vi "ArmControlManager.vi"(0 "Arm Shoulder Manual Control":dbl, 1 "Arm Extend Manual Control":dbl, 3 "Shoulder Sensor Unit Conversion (ticks/rad)":dbl, 4 "Extend Sensor Unit Coversion (ticks/in)":dbl, 5 "Arm Shoulder Motion Profile":T22[](array[typedef]) {"Time (ms)" items=["TrajectoryDuration_0ms"=0, "TrajectoryDuration_5ms"=5, "TrajectoryDuration_10ms"=10, "TrajectoryDuration_20ms"=20, "TrajectoryDuration_30ms"=30, "TrajectoryDuration_40ms"=40, "TrajectoryDuration_50ms"=50, "TrajectoryDuration_100ms"=100]}, 7 "Arm Extend Motion Profile":T22[](array[typedef]) {"Time (ms)" items=["TrajectoryDuration_0ms"=0, "TrajectoryDuration_5ms"=5, "TrajectoryDuration_10ms"=10, "TrajectoryDuration_20ms"=20, "TrajectoryDuration_30ms"=30, "TrajectoryDuration_40ms"=40, "TrajectoryDuration_50ms"=50, "TrajectoryDuration_100ms"=100]}, 8 "ArmCompleteNotifier":refnum<notifier>, 9 "Arm Wrist Motion Profile":T22[](array[typedef]) {"Time (ms)" items=["TrajectoryDuration_0ms"=0, "TrajectoryDuration_5ms"=5, "TrajectoryDuration_10ms"=10, "TrajectoryDuration_20ms"=20, "TrajectoryDuration_30ms"=30, "TrajectoryDuration_40ms"=40, "TrajectoryDuration_50ms"=50, "TrajectoryDuration_100ms"=100]}, 10 "RobotConfig":T1={"Motors"={"DriveRightPrimary"={"CAN Address"=1, "Invert"=FALSE, "InvertSensor"=FALSE, "Unit Conversion Factor"=0.0, "Brake Mode"=enum."Override to Brake", "Reverse Limt Switch Mode"=enum."Normally Closed", "Forward Limt Swith Mode"=enum."Normally Closed", "PWM Channel"=enum."Invalid", "Motor Controller Type"=enum."Talon SRX", "Peak Current (A)"=0, "Continuos Current (A)"=0, "Peak Duration (ms)"=0, "Current Limit Enable"=FALSE}, "DriveRightSecondary"={"CAN Address"=2, "Invert"=FALSE, "InvertSensor"=FALSE, "Unit Conversion Factor"=0.0, "Brake Mode"=enum."Override to Brake", "Reverse Limt Switch Mode"=enum."Normally Closed", "Forward Limt Swith Mode"=enum."Normally Closed", "PWM Channel"=enum."Invalid", "Motor Controller Type"=enum."Talon SRX", "Peak Current (A)"=0, "Continuos Current (A)"=0, "Peak Duration (ms)"=0, "Current Limit Enable"=FALSE}, "DriveLeftPrimary"={"CAN Address"=3, "Invert"=FALSE, "InvertSensor"=FALSE, "Unit Conversion Factor"=0.0, "Brake Mode"=enum."Override to Brake", "Reverse Limt Switch Mode"=enum."Normally Closed", "Forward Limt Swith Mode"=enum."Normally Closed", "PWM Channel"=enum."Invalid", "Motor Controller Type"=enum."Talon SRX", "Peak Current (A)"=0, "Continuos Current (A)"=0, "Peak Duration (ms)"=0, "Current Limit Enable"=FALSE}, "DriveLeftSecondary"={"CAN Address"=4, "Invert"=FALSE, "InvertSensor"=FALSE, "Unit Conversion Factor"=0.0, "Brake Mode"=enum."Override to Brake", "Reverse Limt Switch Mode"=enum."Normally Closed", "Forward Limt Swith Mode"=enum."Normally Closed", "PWM Channel"=enum."Invalid", "Motor Controller Type"=enum."Talon SRX", "Peak Current (A)"=0, "Continuos Current (A)"=0, "Peak Duration (ms)"=0, "Current Limit Enable"=FALSE}, "RearClimb"={"CAN Address"=8, "Invert"=FALSE, "InvertSensor"=FALSE, "Unit Conversion Factor"=0.0, "Brake Mode"=enum."Override to Brake", "Reverse Limt Switch Mode"=enum."Normally Closed", "Forward Limt Swith Mode"=enum."Normally Closed", "PWM Channel"=enum."Invalid", "Motor Controller Type"=enum."Talon SRX", "Peak Current (A)"=0, "Continuos Current (A)"=0, "Peak Duration (ms)"=0, "Current Limit Enable"=FALSE}, "Front Climb"={"CAN Address"=7, "Invert"=FALSE, "InvertSensor"=FALSE, "Unit Conversion Factor"=0.0, "Brake Mode"=enum."Override to Brake", "Reverse Limt Switch Mode"=enum."Normally Closed", "Forward Limt Swith Mode"=enum."Normally Closed", "PWM Channel"=enum."Invalid", "Motor Controller Type"=enum."Talon SRX", "Peak Current (A)"=0, "Continuos Current (A)"=0, "Peak Duration (ms)"=0, "Current Limit Enable"=FALSE}, "Climb Drive"={"CAN Address"=5, "Invert"=FALSE, "InvertSensor"=FALSE, "Unit Conversion Factor"=0.0, "Brake Mode"=enum."Override to Brake", "Reverse Limt Switch Mode"=enum."Normally Closed", "Forward Limt Swith Mode"=enum."Normally Closed", "PWM Channel"=enum."Invalid", "Motor Controller Type"=enum."Talon SRX", "Peak Current (A)"=0, "Continuos Current (A)"=0, "Peak Duration (ms)"=0, "Current Limit Enable"=FALSE}, "Shoulder1"={"CAN Address"=6, "Invert"=FALSE, "InvertSensor"=FALSE, "Unit Conversion Factor"=0.0, "Brake Mode"=enum."Override to Brake", "Reverse Limt Switch Mode"=enum."Normally Closed", "Forward Limt Swith Mode"=enum."Normally Closed", "PWM Channel"=enum."Invalid", "Motor Controller Type"=enum."Talon SRX", "Peak Current (A)"=0, "Continuos Current (A)"=0, "Peak Duration (ms)"=0, "Current Limit Enable"=FALSE}, "Shoulder2"={"CAN Address"=9, "Invert"=FALSE, "InvertSensor"=FALSE, "Unit Conversion Factor"=0.0, "Brake Mode"=enum."Override to Brake", "Reverse Limt Switch Mode"=enum."Normally Closed", "Forward Limt Swith Mode"=enum."Normally Closed", "PWM Channel"=enum."Invalid", "Motor Controller Type"=enum."Talon SRX", "Peak Current (A)"=0, "Continuos Current (A)"=0, "Peak Duration (ms)"=0, "Current Limit Enable"=FALSE}, "Wrist"={"CAN Address"=10, "Invert"=FALSE, "InvertSensor"=FALSE, "Unit Conversion Factor"=0.0, "Brake Mode"=enum."Override to Brake", "Reverse Limt Switch Mode"=enum."Disabled", "Forward Limt Swith Mode"=enum."Disabled", "PWM Channel"=enum."Invalid", "Motor Controller Type"=enum."Talon SRX", "Peak Current (A)"=0, "Continuos Current (A)"=0, "Peak Duration (ms)"=0, "Current Limit Enable"=FALSE}, "Extension"={"CAN Address"=11, "Invert"=FALSE, "InvertSensor"=FALSE, "Unit Conversion Factor"=0.0, "Brake Mode"=enum."Override to Brake", "Reverse Limt Switch Mode"=enum."Disabled", "Forward Limt Swith Mode"=enum."Disabled", "PWM Channel"=enum."Invalid", "Motor Controller Type"=enum."Talon SRX", "Peak Current (A)"=0, "Continuos Current (A)"=0, "Peak Duration (ms)"=0, "Current Limit Enable"=FALSE}, "CargoIntake"={"CAN Address"=11, "Invert"=FALSE, "InvertSensor"=FALSE, "Unit Conversion Factor"=0.0, "Brake Mode"=enum."Override to Brake", "Reverse Limt Switch Mode"=enum."Disabled", "Forward Limt Swith Mode"=enum."Disabled", "PWM Channel"=enum."Invalid", "Motor Controller Type"=enum."Talon SRX", "Peak Current (A)"=0, "Continuos Current (A)"=0, "Peak Duration (ms)"=0, "Current Limit Enable"=FALSE}, "Intake2"={"CAN Address"=11, "Invert"=FALSE, "InvertSensor"=FALSE, "Unit Conversion Factor"=0.0, "Brake Mode"=enum."Override to Brake", "Reverse Limt Switch Mode"=enum."Disabled", "Forward Limt Swith Mode"=enum."Disabled", "PWM Channel"=enum."Invalid", "Motor Controller Type"=enum."Talon SRX", "Peak Current (A)"=0, "Continuos Current (A)"=0, "Peak Duration (ms)"=0, "Current Limit Enable"=FALSE}}, "Sensors"={"IMU"={"Yaw Axis"=enum."Z", "SPI Bus"=enum."SPI MXP", "AHRS Algorithm"=enum."Complementary", "Calibration Time (s)"=3.0, "Calibrate On Open"=TRUE}, "HomingButton"={"DIOChannel"=enum."DIO 0", "Active Low"=FALSE}, "HomingLED_Green"={"DIOChannel"=enum."DIO 0", "Active Low"=FALSE}, "HomingLED_Yellow"={"DIOChannel"=enum."DIO 0", "Active Low"=FALSE}, "HomingLED_Red"={"DIOChannel"=enum."DIO 0", "Active Low"=FALSE}}, "PID"={"FrontClimb"={"P"=0.0, "I"=0.0, "D"=0.0, "F"=0.0, "IZone"=0.0}, "RearClimb"={"P"=0.0, "I"=0.0, "D"=0.0, "F"=0.0, "IZone"=0.0}, "ArmShoulder"={"P"=0.0, "I"=0.0, "D"=0.0, "F"=0.0, "IZone"=0.0}, "ArmExtend"={"P"=0.0, "I"=0.0, "D"=0.0, "F"=0.0, "IZone"=0.0}, "ArmWrist"={"P"=0.0, "I"=0.0, "D"=0.0, "F"=0.0, "IZone"=0.0}}, "Solenoids"={" Shifter"={"SolenoidChannel"=enum."Solenoid 3", "Invert"=FALSE}, "Hatch Grip"={"SolenoidChannel"=enum."Solenoid 0", "Invert"=FALSE}, "Hatch Extend"={"SolenoidChannel"=enum."Solenoid 0", "Invert"=FALSE}, "Manipulator Slide"={"SolenoidChannel"=enum."Solenoid 0", "Invert"=FALSE}, "Hatch Floor Intake"={"SolenoidChannel"=enum."Solenoid 0", "Invert"=FALSE}}, "Enable Compressor"=TRUE, "MotionMagic"={"FrontClimbExtend"={"CruiseVelocity"=0, "Acceleration"=0}, "RearClimbExtend"={"CruiseVelocity"=0, "Acceleration"=0}, "FrontClimbRetract"={"CruiseVelocity"=0, "Acceleration"=0}, "RearClimbRetract"={"CruiseVelocity"=0, "Acceleration"=0}}, "RobotDimensions"={"Length (in)"=0.0, "Shoulder Height (in)"=0.0, "Frame Height (in)"=0.0, "Arm Center to Front of Robot (in)"=0.0, "Arm Min Extension (in)"=0.0, "Arm Max Extension (in)"=0.0}, "Arm Home Position"={"Radius (in)"=0.0, "ShoulderAngle (rad)"=0.0, "WristAngle (rad)"=0.0}, "Climb Home Position"={"Back Climb"=0.0, "Front Climb"=0.0}, "Climb Positions"={"Retract"=0.0, "Level 2"=0.0, "Level 3"=0.0}}, 11 "arm homing state":T25, 12 "Arm Extend Motor DevRef":T19={"DeviceStatus"={"status"=FALSE, "code"=0, "source"=""}, "Type"=enum."PWM", "PWM"={"PWM Channel"=enum."PWM 1", "DeadBand"={"Name"="", "maxPositivePwm"=0, "minPositivePwm"=0, "centerPwm"=0, "maxNegativePwm"=0, "minNegativePwm"=0, "angularRange"=0}}, "CAN"={"Device Number"=0, "SetOutput VI Ref"=variant(enum8{"Percent VBus", "Current", "Speed", "Position", "Voltage"} enum."Percent VBus"), "GetOutput VI Ref"=variant(refnum<k1> refnum), "Enable VI Ref"=variant(dbl 12.0), "Disable VI Ref"=variant(enum8{"Percent VBus", "Speed", "Position", "Slave", "Unchanged / Invalid", "Voltage Compensation", "Current", "Motion Profile"} enum."Percent VBus"), "Data"=variant}, "Invert"=FALSE, "DIO PWM"={"PWM \"Enable\" Channel"=enum."Invalid", "DIOChannel"=enum."Invalid", "PWM Rate"=0.0}}, 13 "New Motion Profile":bool, 14 "Arm Shoulder Motor DevRef":T19={"DeviceStatus"={"status"=FALSE, "code"=0, "source"=""}, "Type"=enum."PWM", "PWM"={"PWM Channel"=enum."PWM 1", "DeadBand"={"Name"="", "maxPositivePwm"=0, "minPositivePwm"=0, "centerPwm"=0, "maxNegativePwm"=0, "minNegativePwm"=0, "angularRange"=0}}, "CAN"={"Device Number"=0, "SetOutput VI Ref"=variant(enum8{"Percent VBus", "Current", "Speed", "Position", "Voltage"} enum."Percent VBus"), "GetOutput VI Ref"=variant(refnum<k1> refnum), "Enable VI Ref"=variant(dbl 12.0), "Disable VI Ref"=variant(enum8{"Percent VBus", "Speed", "Position", "Slave", "Unchanged / Invalid", "Voltage Compensation", "Current", "Motion Profile"} enum."Percent VBus"), "Data"=variant}, "Invert"=FALSE, "DIO PWM"={"PWM \"Enable\" Channel"=enum."Invalid", "DIOChannel"=enum."Invalid", "PWM Rate"=0.0}}, 15 "Arm Wrist Manual Control":dbl, 16 "Arm Wrist Motor DevRef":T19={"DeviceStatus"={"status"=FALSE, "code"=0, "source"=""}, "Type"=enum."PWM", "PWM"={"PWM Channel"=enum."PWM 1", "DeadBand"={"Name"="", "maxPositivePwm"=0, "minPositivePwm"=0, "centerPwm"=0, "maxNegativePwm"=0, "minNegativePwm"=0, "angularRange"=0}}, "CAN"={"Device Number"=0, "SetOutput VI Ref"=variant(enum8{"Percent VBus", "Current", "Speed", "Position", "Voltage"} enum."Percent VBus"), "GetOutput VI Ref"=variant(refnum<k1> refnum), "Enable VI Ref"=variant(dbl 12.0), "Disable VI Ref"=variant(enum8{"Percent VBus", "Speed", "Position", "Slave", "Unchanged / Invalid", "Voltage Compensation", "Current", "Motion Profile"} enum."Percent VBus"), "Data"=variant}, "Invert"=FALSE, "DIO PWM"={"PWM \"Enable\" Channel"=enum."Invalid", "DIOChannel"=enum."Invalid", "PWM Rate"=0.0}}, 17 "Wrist Sensor Unit Coversion (ticks/rad)":dbl) -> (20 "Arm Control State":T24, 25 "Sensor Reset Detected":bool)   [LabVIEW 2018]
uses:
  General/MotionProfiling/TypeDefs/TrajectoryPoint.ctl
  <vilib>/Rock Robotics/WPI/ThirdParty/Phoenix-LabVIEW/Motor Controller/Controls/CTRE_Phoenix_MotorControl_TrajectoryPointTimeDur.ctl
  General/MotionProfiling/TypeDefs/MotionProfileControlState.ctl
  <vilib>/Rock Robotics/WPI/MotorControl/WPI_MotorControlDeviceRef.ctl
  <vilib>/Rock Robotics/WPI/MotorControl/WPI_MotorControlType.ctl
  <vilib>/Rock Robotics/SystemInterfaces/DIO/FPGA_DIOPWMChannel.ctl
  <vilib>/Rock Robotics/WPI/PWM/WPI_PWMDeadband.ctl
  <vilib>/Rock Robotics/SystemInterfaces/DIO/FPGA_DIOChannel.ctl
  General/MotionProfiling/TypeDefs/MPSendState.ctl
  TypeDefs/ConfigComponents/Config_Robot.ctl
  ArgosLib/Config/ConfigComponents/TypeDefs/Config_Motor.ctl
  <vilib>/Rock Robotics/WPI/ThirdParty/Phoenix-LabVIEW/Motor Controller/Controls/CTRE_Phoenix_MotorControl_NeutralMode.ctl
  <vilib>/Rock Robotics/WPI/ThirdParty/Phoenix-LabVIEW/Motor Controller/Controls/CTRE_Phoenix_MotorControl_LimitSwitchNormal.ctl
  ArgosLib/Config/ConfigComponents/TypeDefs/Config_MotorCtrlType.ctl
  ArgosLib/Config/ConfigComponents/TypeDefs/Config_IMU.ctl
  <vilib>/Rock Robotics/SystemInterfaces/spilib/spi_bus.ctl
  ArgosLib/Config/ConfigComponents/TypeDefs/Config_DigitalIO.ctl
  ArgosLib/Config/ConfigComponents/TypeDefs/Config_PIDParams.ctl
  ArgosLib/Config/ConfigComponents/TypeDefs/Config_SingleSolenoid.ctl
  <vilib>/Rock Robotics/WPI/Solenoid/WPI_SolenoidChannel.ctl
  ArgosLib/Config/ConfigComponents/TypeDefs/Config_MotionMagicParams.ctl
  TypeDefs/ConfigComponents/Config_Dimensions.ctl
  TypeDefs/ArmCoordinate.ctl
  Climber/TypeDefs/ClimberPositionHeights.ctl
  TypeDefs/ArmHomingState.ctl
  ArgosLib/Signal Processing/TypeDefs/EdgeDetector_Type.ctl
  <vilib>/Rock Robotics/WPI/DriverStation/WPI_DriverStationRobotMode2.ctl
  TypeDefs/ArmAbsolutePosition.ctl
  <vilib>/Rock Robotics/WPI/ThirdParty/Phoenix-LabVIEW/Motor Controller/Controls/CTRE_Phoenix_MotorControl_ControlMode.ctl
  Global_Var-RefNum/MotionProfileControlData.vi
  <vilib>/Rock Robotics/WPI/ThirdParty/Phoenix-LabVIEW/Motor Controller/Get/CTRE_Phoenix_MotorController_GetSelectedSensorData.vi
  Global_Var-RefNum/DriversStationData.vi
  <vilib>/Rock Robotics/WPI/ThirdParty/Phoenix-LabVIEW/Motor Controller/Get/CTRE_Phoenix_MotorController_GetVoltage.vi
  ArgosLib/ArgosLib.lvlib
panel:
  out "ArmWristV":dbl(graph)
  out "ArmWrist":T18(graph)
  in  "MP State Timeout (ms)":u32
  in  "Tab Control":enum32{"I/O", "Calibration", "Status"}(tab)
  in  "WristErrorThresh (rad)":dbl=0.1745
  in  "ExtendErrorThresh (in)":dbl=3.0
  in  "ShoulderErrorThresh (rad)":dbl=0.1745
  in  "ClearMotionProfile":bool
  in  "StallDetectTime(ms)":u32=200
  in  "EnableStallDetection":bool
  in  "Reset Wrist Rotate Sensor":bool
  in  "Rotate Wrist Position (rad)":dbl
  out "Max Wrist Rotate Speed (Sensor Units per 100 ms)":i32
  in  "Reset Wrist Rotate Max":bool
  out "Max Extend Speed (Sensor Units per 100 ms)":i32
  out "Max Shoulder Rotate Speed (Sensor Units per 100 ms)":i32
  in  "Reset Shoulder Rotate Max":bool
  in  "Reset Extend Max":bool
  in  "Reset Extend Sensor":bool
  in  "Reset Shoulder Rotate Sensor":bool
  in  "Extend Position (in)":dbl=21.5
  in  "Rotate Shoulder Position (rad)":dbl=1.57
  out "WristRotate":T18
  out "WristRotate":T26
  out "WristRotateFaults":T27
  out "MP Send State":T28
  out "ShoulderRotate":T26
  out "Extension":T26
  out "ShoulderRotate":T18
  out "Extension":T18
  out "ExtendFaults":T27
  out "ShoulderRotateFaults":T27
  out "Arm Tracking":cluster{dbl[], dbl[]}[](graph)
  out "ArmShoulderV":dbl(graph)
  out "ArmExtensionV":dbl(graph)
  out "ArmExtension":T18(graph)
  out "ArmShoulder":T18(graph)
  # "10 degrees or 3 inches\nerror for 200ms will\ncancel motion"
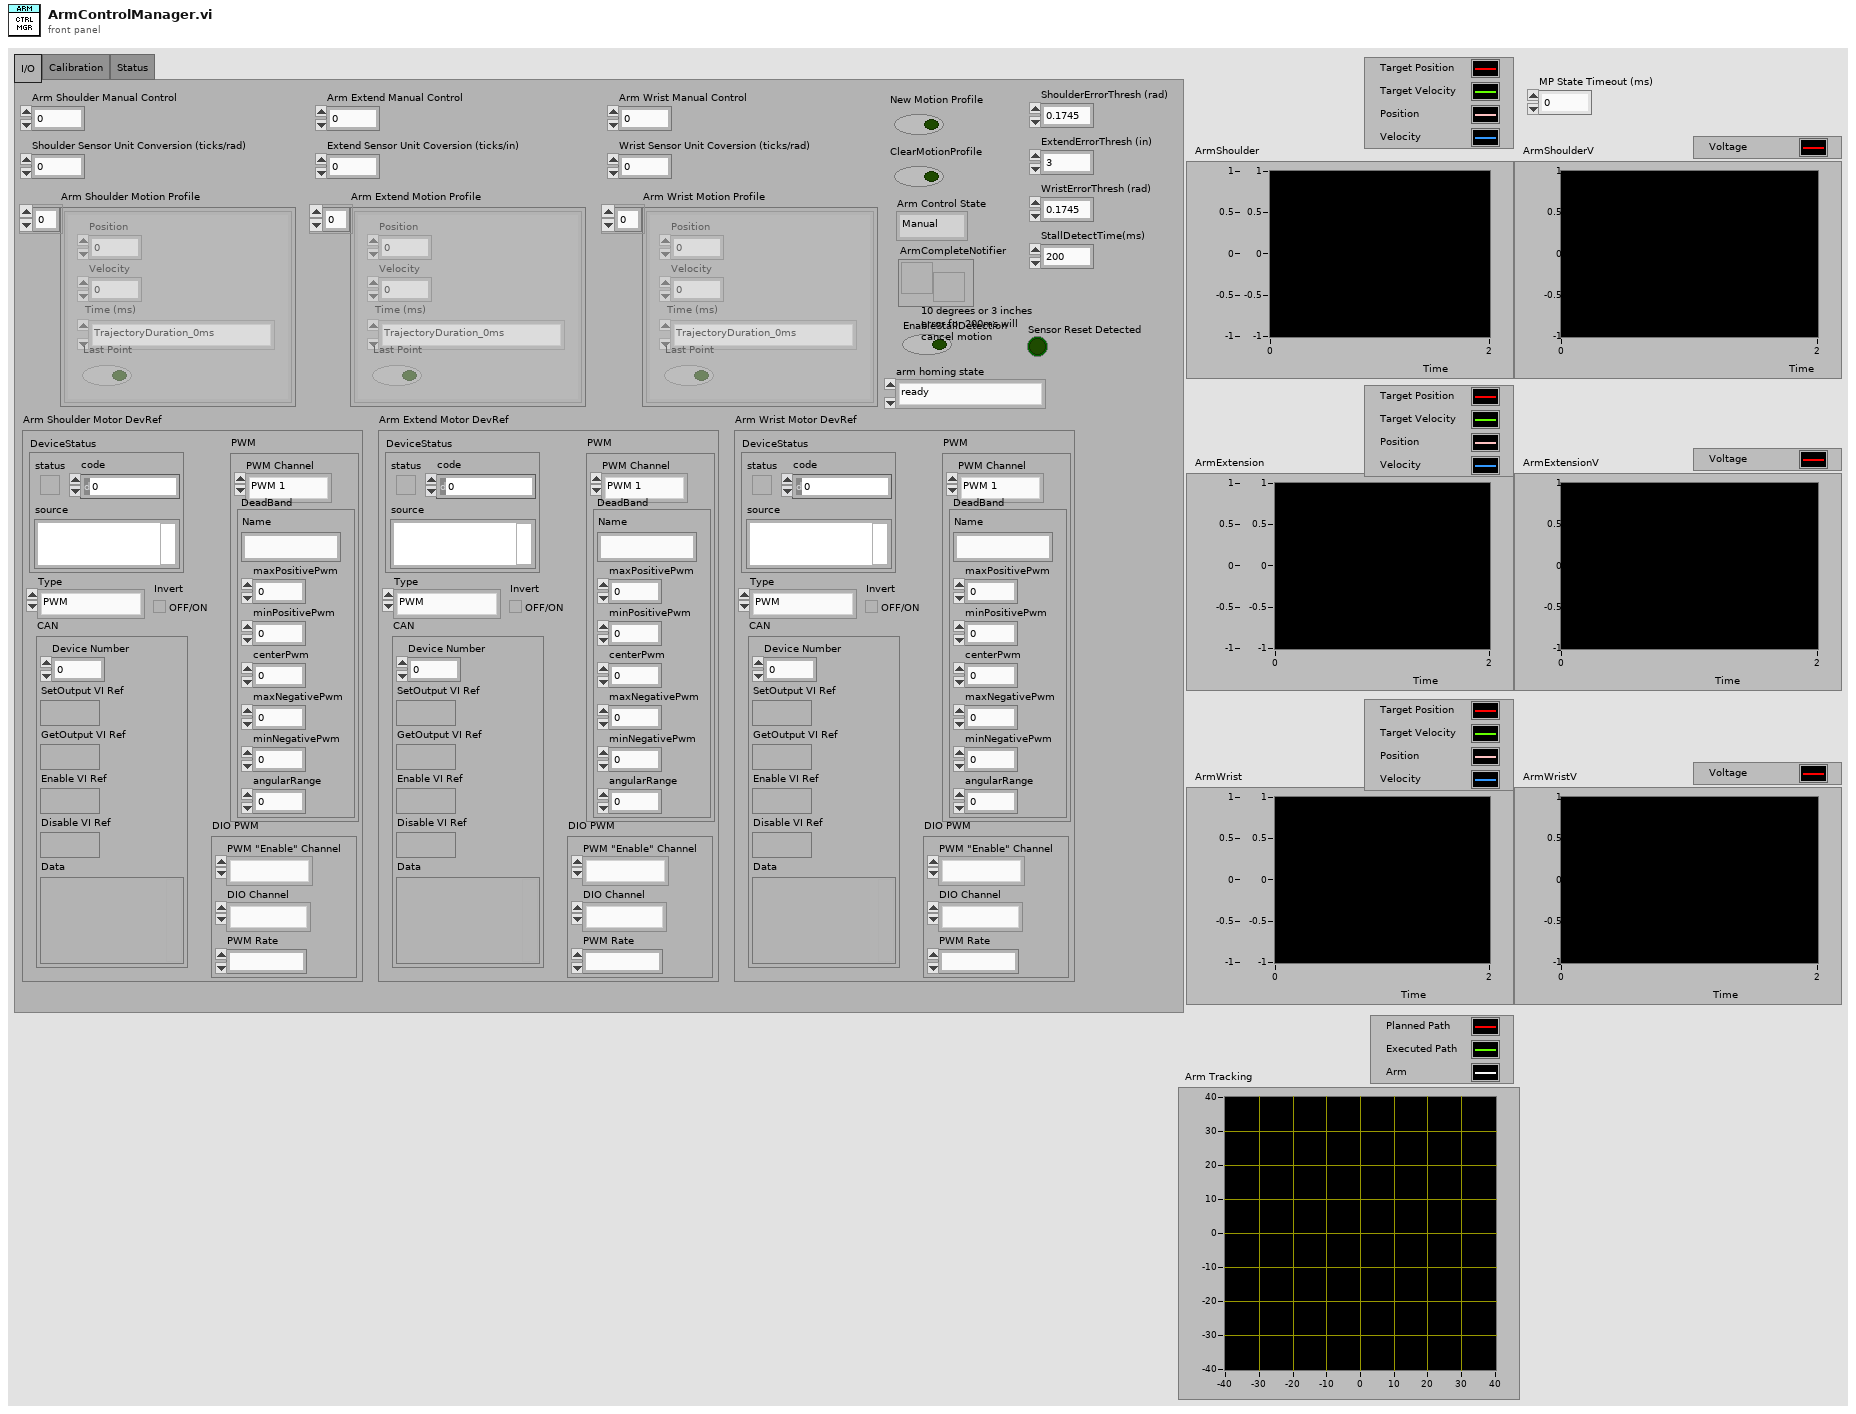
[diagram p1: front panel]
types:
  T1 = typedef "Config_Robot.ctl" = cluster{"Motors":cluster{"DriveRightPrimary":T2, "DriveRightSecondary":T2, "DriveLeftPrimary":T2, "DriveLeftSecondary":T2, "RearClimb":T2, "Front Climb":T2, "Climb Drive":T2, "Shoulder1":T2, "Shoulder2":T2, "Wrist":T2, "Extension":T2, "CargoIntake":T2, "Intake2":T2}, "Sensors":cluster{"IMU":T7, "HomingButton":T9, "HomingLED_Green":T9, "HomingLED_Yellow":T9, "HomingLED_Red":T9}, "PID":cluster{"FrontClimb":T11, "RearClimb":T11, "ArmShoulder":T11, "ArmExtend":T11, "ArmWrist":T11}, "Solenoids":cluster{" Shifter":T12, "Hatch Grip":T12, "Hatch Extend":T12, "Manipulator Slide":T12, "Hatch Floor Intake":T12}, "Enable Compressor":bool, "MotionMagic":cluster{"FrontClimbExtend":T14, "RearClimbExtend":T14, "FrontClimbRetract":T14, "RearClimbRetract":T14}, "RobotDimensions":T15, "Arm Home Position":T16, "Climb Home Position":cluster{"Back Climb":dbl, "Front Climb":dbl}, "Climb Positions":T17}
  T2 = typedef "ArgosLib.lvlib/Config_Motor.ctl" = cluster{"CAN Address":u8, "Invert":bool, "InvertSensor":bool, "Unit Conversion Factor":dbl, "Brake Mode":T3, "Reverse Limt Switch Mode":T4, "Forward Limt Swith Mode":T4, "PWM Channel":T5, "Motor Controller Type":T6, "Peak Current (A)":i32, "Continuos Current (A)":i32, "Peak Duration (ms)":i32, "Current Limit Enable":bool}
  T3 = typedef "CTRE_Phoenix_MotorControl_NeutralMode.ctl" = enum8{"EEPROMSetting", "Override to Coast", "Override to Brake"}
  T4 = typedef "CTRE_Phoenix_MotorControl_LimitSwitchNormal.ctl" = enum16{"Normally Open", "Normally Closed", "Disabled"}
  T5 = typedef "FPGA_DIOPWMChannel.ctl" = enum8{"PWM 0", "PWM 1", "PWM 2", "PWM 3", "PWM 4", "PWM 5", "PWM 6", "PWM 7", "PWM 8", "PWM 9", "PWM MXP 0", "PWM MXP 1", "PWM MXP 2", "PWM MXP 3", "PWM MXP 4", "PWM MXP 5", "PWM MXP 6", "PWM MXP 7", "PWM MXP 8", "PWM MXP 9", "Invalid"}
  T6 = typedef "ArgosLib.lvlib/Config_MotorCtrlType.ctl" = enum16{"Disabled", "Talon SRX", "Talon SR"}
  T7 = typedef "ArgosLib.lvlib/Config_IMU.ctl" = cluster{"Yaw Axis":enum16{"X", "Y", "Z"}, "SPI Bus":T8, "AHRS Algorithm":enum16{"Complementary", "Madgwick"}, "Calibration Time (s)":dbl, "Calibrate On Open":bool}
  T8 = typedef "spi_bus.ctl" = enum16{"SPI On-Board, CS0", "SPI On-Board, CS1", "SPI On-Board, CS2", "SPI On-Board, CS3", "SPI MXP", "Invalid"}
  T9 = typedef "ArgosLib.lvlib/Config_DigitalIO.ctl" = cluster{"DIOChannel":T10, "Active Low":bool}
  T10 = typedef "FPGA_DIOChannel.ctl" = enum8{"DIO 0", "DIO 1", "DIO 2", "DIO 3", "DIO 4", "DIO 5", "DIO 6", "DIO 7", "DIO 8", "DIO 9", "DIO MXP 0", "DIO MXP 1", "DIO MXP 2", "DIO MXP 3", "DIO MXP 4", "DIO MXP 5", "DIO MXP 6", "DIO MXP 7", "DIO MXP 8", "DIO MXP 9", "DIO MXP 10", "DIO MXP 11", "DIO MXP 12", "DIO MXP 13", "DIO MXP 14", "DIO MXP 15", "SPI Port CS1", "SPI Port CS2", "SPI Port CS3", "SPI Port MISO", "SPI Port MOSI", "Invalid"}
  T11 = typedef "ArgosLib.lvlib/Config_PIDParams.ctl" = cluster{"P":dbl, "I":dbl, "D":dbl, "F":dbl, "IZone":dbl}
  T12 = typedef "ArgosLib.lvlib/Config_SingleSolenoid.ctl" = cluster{"SolenoidChannel":T13, "Invert":bool}
  T13 = typedef "WPI_SolenoidChannel.ctl" = enum8{"Solenoid 0", "Solenoid 1", "Solenoid 2", "Solenoid 3", "Solenoid 4", "Solenoid 5", "Solenoid 6", "Solenoid 7", "Invalid"}
  T14 = typedef "Config_MotionMagicParams.ctl" = cluster{"CruiseVelocity":i32, "Acceleration":i32}
  T15 = typedef "Config_Dimensions.ctl" = cluster{"Length (in)":dbl, "Shoulder Height (in)":dbl, "Frame Height (in)":dbl, "Arm Center to Front of Robot (in)":dbl, "Arm Min Extension (in)":dbl, "Arm Max Extension (in)":dbl}
  T16 = typedef "ArmCoordinate.ctl" = cluster{"Radius (in)":dbl, "ShoulderAngle (rad)":dbl, "WristAngle (rad)":dbl}
  T17 = typedef "ClimberPositionHeights.ctl" = cluster{"Retract":dbl, "Level 2":dbl, "Level 3":dbl}
  T18 = cluster{"Position (Sensor Units)":i32, "Velocity (Sensor Units per 100 ms)":i32, "Position (Raw Sensor Units)":i32, "Velocity (Raw Sensor Units per 100 ms)":i32}
  T19 = typedef "WPI_MotorControlDeviceRef.ctl" = cluster{"DeviceStatus":errorcluster, "Type":T20, "PWM":cluster{"PWM Channel":T5, "DeadBand":T21}, "CAN":cluster{"Device Number":u8, "SetOutput VI Ref":variant, "GetOutput VI Ref":variant, "Enable VI Ref":variant, "Disable VI Ref":variant, "Data":variant}, "Invert":bool, "DIO PWM":cluster{"PWM \"Enable\" Channel":T5, "DIOChannel":T10, "PWM Rate":dbl}}
  T20 = typedef "WPI_MotorControlType.ctl" = enum16{"PWM", "CAN", "DIO PWM"}
  T21 = typedef "WPI_PWMDeadband.ctl" = cluster{"Name":string, "maxPositivePwm":i32, "minPositivePwm":i32, "centerPwm":i32, "maxNegativePwm":i32, "minNegativePwm":i32, "angularRange":u16}
  T22 = typedef "TrajectoryPoint.ctl" = cluster{"Position ":dbl, "Velocity ":dbl, "Time (ms)":T23, "Last Point":bool}
  T23 = typedef "CTRE_Phoenix_MotorControl_TrajectoryPointTimeDur.ctl" = i32
  T24 = typedef "MotionProfileControlState.ctl" = enum16{"Manual", "Auto_Idle", "Auto_Run"}
  T25 = typedef "ArmHomingState.ctl" = enum16{"ready", "homing in progress", "homing complete ", "homing failed"}
  T26 = cluster{"Top Buffer Remaining":i32, "Top Buffer Count":i32, "Bottom Buffer Count":i32, "Has Underrun?":bool, "Is Underrun?":bool, "Active Point Valid?":bool, "Is Last?":bool, "Profile Slot Select 0":i32, "Output Enable":i32, "Time Duration (ms)":i32, "Profile Slot Select 1":i32}
  T27 = cluster{"Under Voltage":bool, "Forward Limit Switch":bool, "Reverse Limit Switch":bool, "Forward Soft Limit":bool, "Reverse Soft Limit":bool, "Hardware Failure":bool, "Reset During Enable":bool, "Sensor Overflow":bool, "Sensor Out of Phase":bool, "Hardware ESD Reset":bool, "Remote Loss of Signal":bool}
  T28 = typedef "MPSendState.ctl" = enum16{"Disable", "Commit Points", "Enable", "Done", "Failed"}
  T29 = typedef "ArgosLib.lvlib/EdgeDetector_Type.ctl" = enum16{"RisingEdge", "FallingEdge", "Both"}
  T30 = typedef "ArmAbsolutePosition.ctl" = cluster{"X (in)":dbl, "Y (in)":dbl, "Wrist (rad)":dbl}
  T31 = typedef "WPI_DriverStationRobotMode2.ctl" = enum16{"Autonomous Disabled", "Autonomous Enabled", "Teleop Disabled", "Teleop Enabled", "Disconnected", "Finish", "Test Disabled", "Test Enabled", "Emergency Stopped"}
  T32 = cluster{"Position (Sensor Units)":i32, "Velocity (Sensor Units per 100 ms)":i32, "Position (Raw Sensor Units)":i32, "Velocity (Raw Sensor Units per 100 ms)":i32}[]
  T33 = typedef "CTRE_Phoenix_MotorControl_ControlMode.ctl" = u16
  T34 = typedef "ArmMotionProfileControl.ctl" = cluster{"ControlMutex":T35, "Trajectory Points":T22[], "CurrentIndex":u32}
  T35 = typedef "Semaphore RefNum" = refnum<k1>
  T36 = cluster{"Position (Sensor Units)":i32, "Velocity (Sensor Units per 100 ms)":i32, "Position (Raw Sensor Units)":i32, i32}
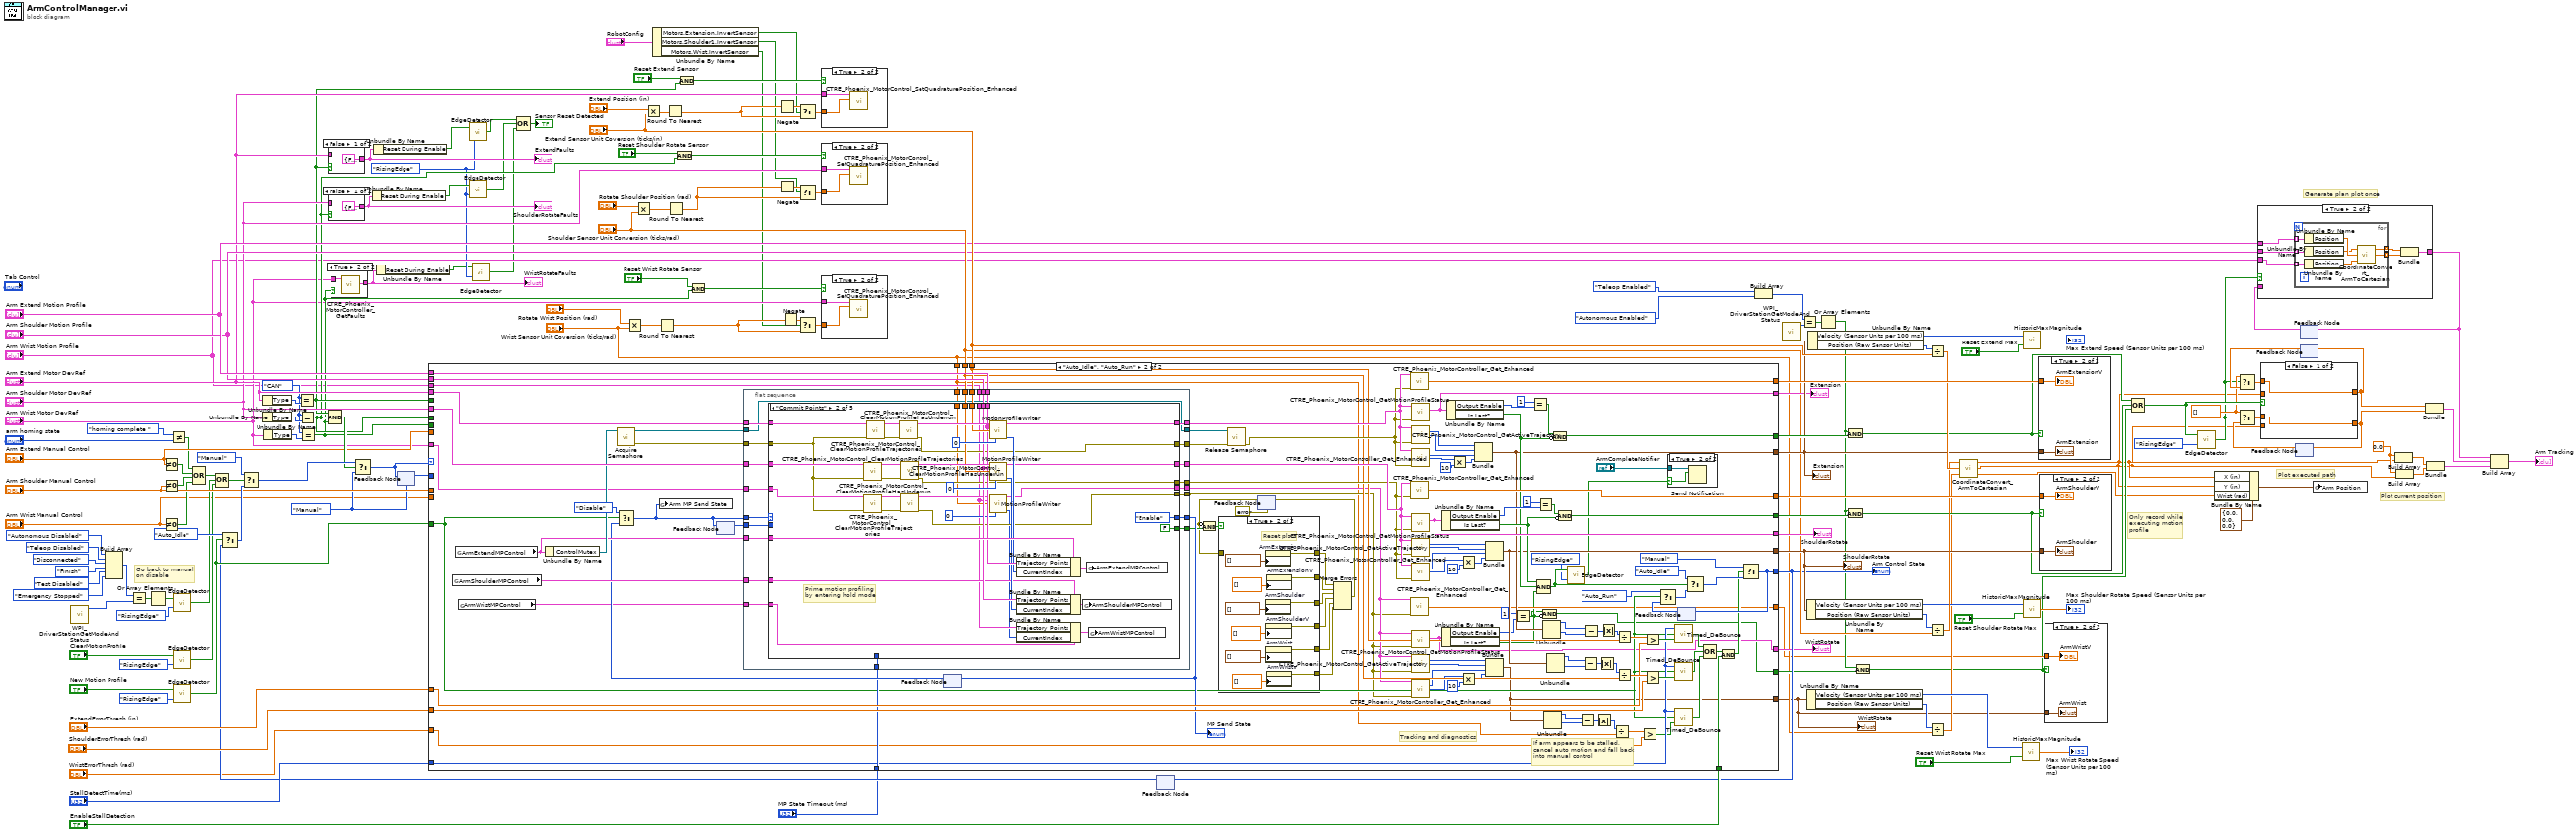
[diagram p0: block diagram]
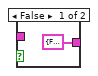
[diagram p3: hidden frame]
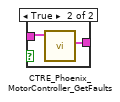
[diagram p5: hidden frame]
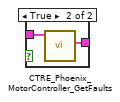
[diagram p6: hidden frame]
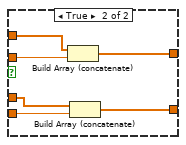
[diagram p8: hidden frame]
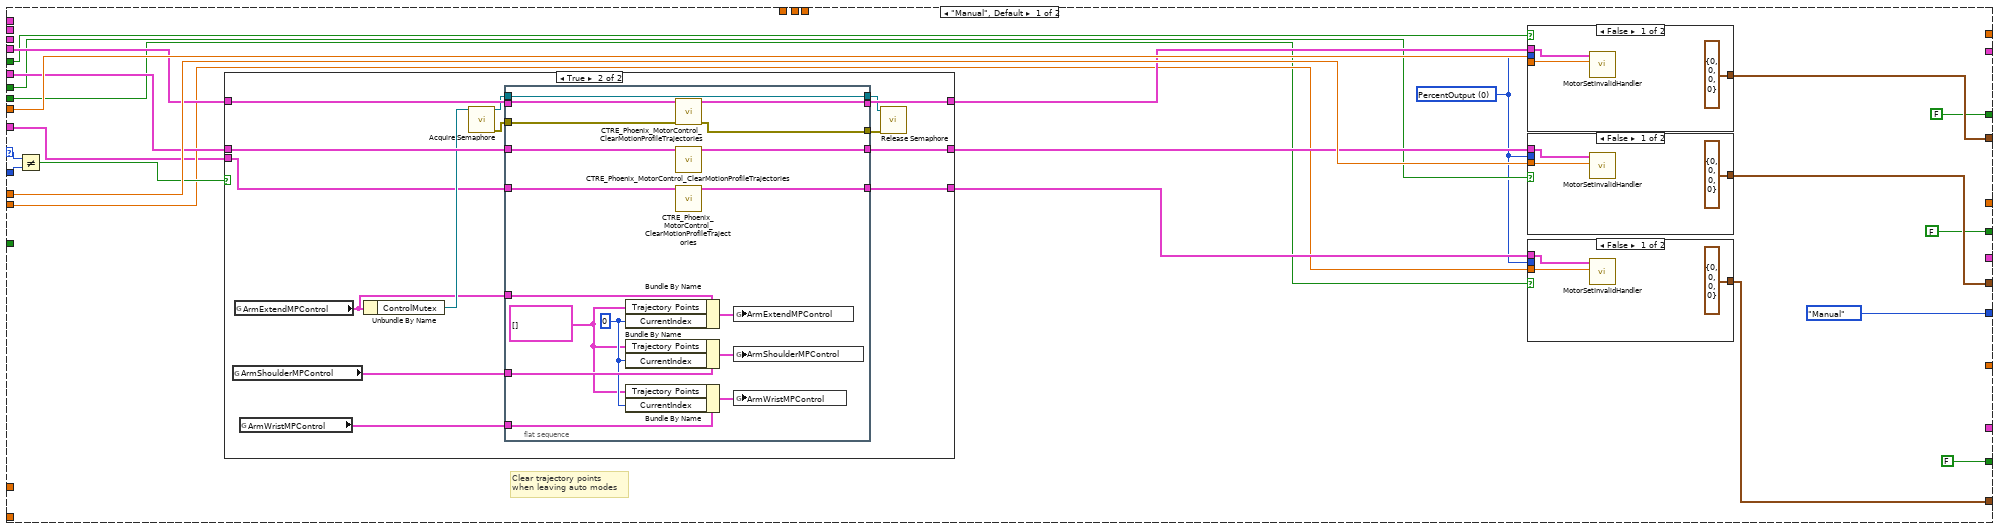
[diagram p13: hidden frame]
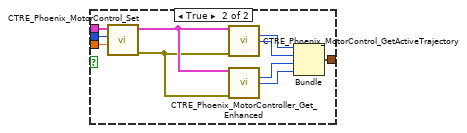
[diagram p14: hidden frame]
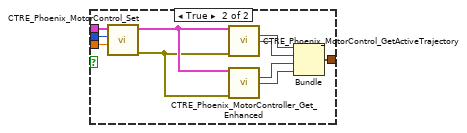
[diagram p15: hidden frame]
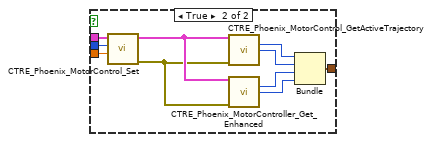
[diagram p16: hidden frame]
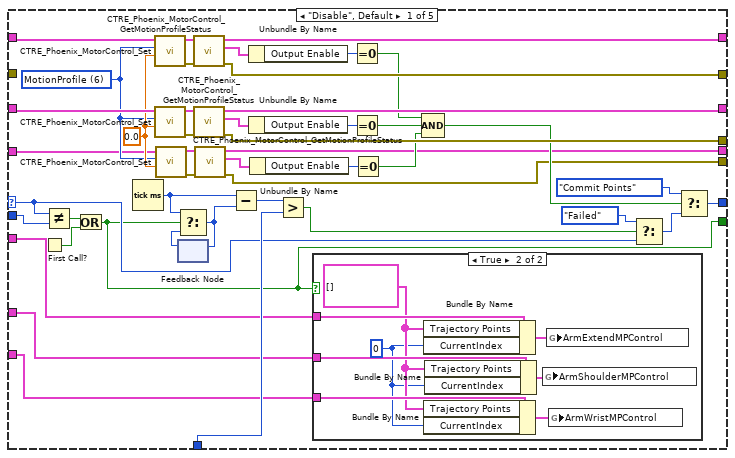
[diagram p20: hidden frame]
diagram:
  w7 = EdgeDetector_Type."RisingEdge" ("DetectorType")
  w64 = MotionProfileControlState."Manual" ("t")
  w55 = WPI_MotorControlType."CAN" ("x")
  w89 = dbl[] [] ("t")
  w123 = 0.0 ("element")
  # "Plot current position"
  # "Plot executed path"
  # "Generate plan plot once"
  # "Go back to manual\non disable"
  # "Only record while\nexecuting motion\nprofile"
  n1 = call <vilib>:"WPI_DriverStationGetModeAndStatus.vi"() -> ("Robot Mode"=w115:T31)  [unwired: 10 in, 1 out]
  n2 = Build Array(WPI_DriverStationRobotMode2."Autonomous Disabled" ("Robot Mode"), WPI_DriverStationRobotMode2."Teleop Disabled" ("Robot Mode"), WPI_DriverStationRobotMode2."Disconnected" ("Robot Mode"), WPI_DriverStationRobotMode2."Finish" ("Robot Mode"), WPI_DriverStationRobotMode2."Test Disabled" ("Robot Mode"), WPI_DriverStationRobotMode2."Emergency Stopped" ("Robot Mode")) -> (w116:T31[])
  n3 = Equal?(x=w116, y=w115) -> (x = y?=w114:bool[])
  n4 = Or Array Elements(Boolean array=w114) -> (logical OR=w113:bool)
  n5 = Not Equal To 0?(x="Arm Extend Manual Control") -> (x != 0?=w156:bool)
  n6 = Not Equal To 0?(x="Arm Shoulder Manual Control") -> (x != 0?=w155:bool)
  n7 = Not Equal To 0?(x="Arm Wrist Manual Control") -> (x != 0?=w59:bool)
  n8 = Not Equal?(x=ArmHomingState."homing complete " ("arm homing state"), y="arm homing state") -> (x != y?=w15:bool)
  n9 = call "EdgeDetector.vi"("DetectorType"=EdgeDetector_Type."RisingEdge", "Input"=w113) -> ("Edge"=w110:bool)
  n10 = call "EdgeDetector.vi"("DetectorType"=EdgeDetector_Type."RisingEdge", "Input"="ClearMotionProfile") -> ("Edge"=w111:bool)
  n11 = call "EdgeDetector.vi"("DetectorType"=EdgeDetector_Type."RisingEdge", "Input"="New Motion Profile") -> ("Edge"=w149:bool)
  n12 = Compound Arithmetic op=OR(w15, w156, w155, w59) -> (w139:bool)
  n13 = Compound Arithmetic op=OR(w139, w110, w111) -> (w140:bool)
  n14 = Unbundle By Name("Arm Extend Motor DevRef") -> ("Type"=w68:T20)
  n15 = Unbundle By Name("Arm Shoulder Motor DevRef") -> ("Type"=w67:T20)
  n16 = Unbundle By Name("Arm Wrist Motor DevRef") -> ("Type"=w56:T20)
  n17 = Equal?(x=w55, y=w68) -> (x = y?=w50:bool)
  n18 = Equal?(x=w55, y=w67) -> (x = y?=w49:bool)
  n19 = Equal?(x=w55, y=w56) -> (x = y?=w48:bool)
  n20 = case shown="False" w50 {
    tunnel: [T27 {"Under Voltage"=FALSE, "Forward Limit Switch"=FALSE, "Reverse Limit Switch"=FALSE, "Forward Soft Limit"=FALSE, "Reverse Soft Limit"=FALSE, "Hardware Failure"=FALSE, "Reset During Enable"=FALSE, "Sensor Overflow"=FALSE, "Sensor Out of Phase"=FALSE, "Hardware ESD Reset"=FALSE, "Remote Loss of Signal"=FALSE} ("Faults") w159] -> w13
    tunnel: "Arm Extend Motor DevRef" -> [_ w158]
    frame False {
    }
    frame True {
      n21 = call <vilib>:"CTRE_Phoenix_MotorController_GetFaults.vi"("PhoenixMotorControlDevRef"=w158) -> ("Faults"=w159:T27)  [unwired: 8 in, 2 out]
    }
  }
  "ExtendFaults" <- w13
  n22 = case shown="False" w49 {
    tunnel: [T27 {"Under Voltage"=FALSE, "Forward Limit Switch"=FALSE, "Reverse Limit Switch"=FALSE, "Forward Soft Limit"=FALSE, "Reverse Soft Limit"=FALSE, "Hardware Failure"=FALSE, "Reset During Enable"=FALSE, "Sensor Overflow"=FALSE, "Sensor Out of Phase"=FALSE, "Hardware ESD Reset"=FALSE, "Remote Loss of Signal"=FALSE} ("Faults") w162] -> w12
    tunnel: "Arm Shoulder Motor DevRef" -> [_ w161]
    frame False {
    }
    frame True {
      n23 = call <vilib>:"CTRE_Phoenix_MotorController_GetFaults.vi"("PhoenixMotorControlDevRef"=w161) -> ("Faults"=w162:T27)  [unwired: 8 in, 2 out]
    }
  }
  "ShoulderRotateFaults" <- w12
  n24 = Compound Arithmetic op=AND(w50, w49, w48) -> (w63:bool)
  n25 = case shown="True" w48 {
    tunnel: [T27 {"Under Voltage"=FALSE, "Forward Limit Switch"=FALSE, "Reverse Limit Switch"=FALSE, "Forward Soft Limit"=FALSE, "Reverse Soft Limit"=FALSE, "Hardware Failure"=FALSE, "Reset During Enable"=FALSE, "Sensor Overflow"=FALSE, "Sensor Out of Phase"=FALSE, "Hardware ESD Reset"=FALSE, "Remote Loss of Signal"=FALSE} ("Faults") w165] -> w14
    tunnel: "Arm Wrist Motor DevRef" -> [_ w164]
    frame False {
    }
    frame True {
      n26 = call <vilib>:"CTRE_Phoenix_MotorController_GetFaults.vi"("PhoenixMotorControlDevRef"=w164) -> ("Faults"=w165:T27)  [unwired: 8 in, 2 out]
    }
  }
  "WristRotateFaults" <- w14
  n27 = Unbundle By Name(w12) -> ("Reset During Enable"=w9:bool)
  n28 = Unbundle By Name(w13) -> ("Reset During Enable"=w11:bool)
  n29 = Unbundle By Name(w14) -> ("Reset During Enable"=w6:bool)
  n30 = feedback #1(w64) -> (w73:T24)
  n31 = call "EdgeDetector.vi"("DetectorType"=w7, "Input"=w11) -> ("Edge"=w10:bool)
  n32 = call "EdgeDetector.vi"("DetectorType"=w7, "Input"=w9) -> ("Edge"=w8:bool)
  n33 = call "EdgeDetector.vi"("DetectorType"=w7, "Input"=w6) -> ("Edge"=w5:bool)
  n34 = Compound Arithmetic op=OR(w10, w8, w5) -> (→"Sensor Reset Detected":bool)
  n35 = Multiply(x="Rotate Wrist Position (rad)", y="Wrist Sensor Unit Coversion (ticks/rad)") -> (x*y=w54:dbl)
  n36 = Multiply(x="Rotate Shoulder Position (rad)", y="Shoulder Sensor Unit Conversion (ticks/rad)") -> (x*y=w126:dbl)
  n37 = Multiply(x="Extend Position (in)", y="Extend Sensor Unit Coversion (ticks/in)") -> (x*y=w128:dbl)
  n38 = Unbundle By Name("RobotConfig") -> ("Motors.Extension.InvertSensor"=w3:bool, "Motors.Shoulder1.InvertSensor"=w2:bool, "Motors.Wrist.InvertSensor"=w1:bool)
  n39 = Round To Nearest(number=w54) -> (nearest integer value=w27:dbl)
  n40 = Round To Nearest(number=w128) -> (nearest integer value=w28:dbl)
  n41 = Round To Nearest(number=w126) -> (nearest integer value=w29:dbl)
  n42 = And(x="Reset Shoulder Rotate Sensor", y=w49) -> (x .and. y?=w61:bool)
  n43 = And(x="Reset Extend Sensor", y=w50) -> (x .and. y?=w62:bool)
  n44 = And(x="Reset Wrist Rotate Sensor", y=w48) -> (x .and. y?=w52:bool)
  n45 = Negate(x=w28) -> (-x=w24:dbl)
  n46 = Negate(x=w29) -> (-x=w25:dbl)
  n47 = Negate(x=w27) -> (-x=w26:dbl)
  n48 = Select(t=w24, s=w3, f=w28) -> (s? t:f=w32:dbl)
  n49 = Select(t=w25, s=w2, f=w29) -> (s? t:f=w31:dbl)
  n50 = Select(t=w26, s=w1, f=w27) -> (s? t:f=w30:dbl)
  n51 = case shown="True" w62 {
    tunnel: "Arm Extend Motor DevRef" -> [_ w167]
    tunnel: w32 -> [_ w166]
    frame False {
    }
    frame True {
      n52 = call <vilib>:"CTRE_Phoenix_MotorControl_SetQuadraturePosition_Enhanced.vi"("New Position"=w166, "PhoenixMotorControlDevRef"=w167) -> ()  [unwired: 8 in, 2 out]
    }
  }
  n53 = case shown="True" w61 {
    tunnel: "Arm Shoulder Motor DevRef" -> [_ w169]
    tunnel: w31 -> [_ w168]
    frame False {
    }
    frame True {
      n54 = call <vilib>:"CTRE_Phoenix_MotorControl_SetQuadraturePosition_Enhanced.vi"("New Position"=w168, "PhoenixMotorControlDevRef"=w169) -> ()  [unwired: 8 in, 2 out]
    }
  }
  n55 = case shown="True" w52 {
    tunnel: "Arm Wrist Motor DevRef" -> [_ w171]
    tunnel: w30 -> [_ w170]
    frame False {
    }
    frame True {
      n56 = call <vilib>:"CTRE_Phoenix_MotorControl_SetQuadraturePosition_Enhanced.vi"("New Position"=w170, "PhoenixMotorControlDevRef"=w171) -> ()  [unwired: 8 in, 2 out]
    }
  }
  n57 = feedback #2() -> (w72:T24)  [unwired: 1 in]
  n58 = Select(t=MotionProfileControlState."Auto_Idle", s=w149, f=w72) -> (s? t:f=w153:T24)
  n59 = Select(t=MotionProfileControlState."Manual" ("Arm Control State"), s=w140, f=w153) -> (s? t:f=w66:T24)
  n60 = Select(t=w66, s=w63, f=w64) -> (s? t:f=w65:T24)
  n61 = feedback-in #1(w65) -> ()
  n62 = case shown="\"Auto_Idle\", \"Auto_Run\"" w65 {
    selector: w65 -> [w193 _]
    tunnel: "Arm Extend Motor DevRef" -> [w185 w348]
    tunnel: "Arm Shoulder Motor DevRef" -> [w184 w347]
    tunnel: "Arm Extend Manual Control" -> [w186 _]
    tunnel: "Arm Shoulder Manual Control" -> [w194 _]
    tunnel: w73 -> [w192 _]
    tunnel: w149 -> [_ w298]
    tunnel: "Arm Extend Motion Profile" -> [_ w350]
    tunnel: "Arm Shoulder Motion Profile" -> [_ w349]
    tunnel: [MotionProfileControlState."Manual" ("Arm Control State") w353] -> w74
    tunnel: [w190 w338] -> w125
    tunnel: [w189 w337] -> w124
    tunnel: [FALSE w379] -> w143
    tunnel: [FALSE w375] -> w145
    tunnel: [_ w368] -> w142
    tunnel: [_ w367] -> w141
    tunnel: "Extend Sensor Unit Coversion (ticks/in)" -> [_ w328]
    tunnel: "Shoulder Sensor Unit Conversion (ticks/rad)" -> [_ w326]
    tunnel: [_ w363] -> w103
    tunnel: [_ w362] -> w102
    tunnel: "ExtendErrorThresh (in)" -> [_ w358]
    tunnel: "ShoulderErrorThresh (rad)" -> [_ w359]
    tunnel: "StallDetectTime(ms)" -> [_ w300]
    tunnel: "EnableStallDetection" -> [_ w330]
    tunnel: "MP State Timeout (ms)" -> [_ w315]
    tunnel: w50 -> [w180 _]
    tunnel: w49 -> [w179 _]
    tunnel: "Arm Wrist Manual Control" -> [w177 _]
    tunnel: "Wrist Sensor Unit Coversion (ticks/rad)" -> [_ w275]
    tunnel: "Arm Wrist Motion Profile" -> [_ w287]
    tunnel: w48 -> [w172 _]
    tunnel: [w175 w269] -> w23
    tunnel: [_ w283] -> w47
    tunnel: [FALSE w270] -> w46
    tunnel: "Arm Wrist Motor DevRef" -> [w173 w289]
    tunnel: "WristErrorThresh (rad)" -> [_ w276]
    tunnel: [_ w284] -> w36
    frame "Manual", Default {
      w176 = T33 0 items=["PercentOutput"=0, "Position"=1, "Velocity"=2, "Current"=3, "Follower"=5, "MotionProfile"=6, "MotionMagic"=7, "MotionMagicArc"=8, "MotionProfileArc"=10, "Disabled"=15] ("Control Mode")
      # "Clear trajectory points\nwhen leaving auto modes"
      n63 = Not Equal?(x=w193, y=w192) -> (x != y?=w181:bool)
      n64 = case shown="True" w181 {
        tunnel: w185 -> [w236 w250]
        tunnel: [w236 w249] -> w183
        tunnel: w184 -> [w235 w248]
        tunnel: [w235 w247] -> w182
        tunnel: [w234 w238] -> w178
        tunnel: w173 -> [w234 w237]
        frame False {
        }
        frame True {
          n65 = global read "MotionProfileControlData.vi" "ArmShoulderMPControl"() -> (w242:T34)
          n66 = global read "MotionProfileControlData.vi" "ArmExtendMPControl"() -> (w243:T34)
          n67 = global read "MotionProfileControlData.vi" "ArmWristMPControl"() -> (w239:T34)
          n68 = Unbundle By Name(w243) -> ("ControlMutex"=w245:T35)
          n69 = call <vilib>:"Acquire Semaphore.vi"("semaphore"=w245) -> ("error out"=w246:errorcluster, "semaphore out"=w241:T35)  [unwired: 4 in, 1 out]
          n70 = flat-sequence {
            tunnel: w250 -> [w267]
            tunnel: [w266] -> w249
            tunnel: w248 -> [w265]
            tunnel: [w264] -> w247
            tunnel: w246 -> [w263]
            tunnel: [w262] -> w244
            tunnel: w243 -> [w261]
            tunnel: w242 -> [w257]
            tunnel: w241 -> [w259]
            tunnel: [w259] -> w240
            tunnel: w239 -> [w254]
            tunnel: [w252] -> w238
            tunnel: w237 -> [w251]
            frame #0 {
              w256 = u32 0 ("CurrentIndex")
              w255 = T22[] [] ("Trajectory Points")
              n71 = Bundle By Name(cluster=w261, "Trajectory Points"=w255, "CurrentIndex"=w256) -> (w260:T34)
              n72 = Bundle By Name(cluster=w257, "Trajectory Points"=w255, "CurrentIndex"=w256) -> (w258:T34)
              n73 = Bundle By Name(cluster=w254, "Trajectory Points"=w255, "CurrentIndex"=w256) -> (w253:T34)
              n74 = call <vilib>:"CTRE_Phoenix_MotorControl_ClearMotionProfileTrajectories.vi"("PhoenixMotorControlDevRef"=w267, "error in"=w263) -> ("PhoenixMotorControlDevRef"=w266:T19, "error out"=w262:errorcluster)  [unwired: 12 in]
              n75 = call <vilib>:"CTRE_Phoenix_MotorControl_ClearMotionProfileTrajectories.vi"("PhoenixMotorControlDevRef"=w265) -> ("PhoenixMotorControlDevRef"=w264:T19)  [unwired: 13 in, 1 out]
              n76 = call <vilib>:"CTRE_Phoenix_MotorControl_ClearMotionProfileTrajectories.vi"("PhoenixMotorControlDevRef"=w251) -> ("PhoenixMotorControlDevRef"=w252:T19)  [unwired: 13 in, 1 out]
              n77 = global write "MotionProfileControlData.vi" "ArmExtendMPControl"(w260) -> ()
              n78 = global write "MotionProfileControlData.vi" "ArmShoulderMPControl"(w258) -> ()
              n79 = global write "MotionProfileControlData.vi" "ArmWristMPControl"(w253) -> ()
            }
          }
          n80 = call <vilib>:"Release Semaphore.vi"("error in (no error)"=w244, "semaphore"=w240) -> ()  [unwired: 4 in, 2 out]
        }
      }
      n81 = case shown="False" w180 {
        tunnel: w176 -> [_ w233]
        tunnel: [T18 {"Position (Sensor Units)"=0, "Velocity (Sensor Units per 100 ms)"=0, "Position (Raw Sensor Units)"=0, "Velocity (Raw Sensor Units per 100 ms)"=0} w232] -> w190
        tunnel: w186 -> [w222 w225]
        tunnel: w183 -> [w223 w224]
        frame False {
          n82 = call "MotorSetInvalidHandler.vi"("Output"=w222, "MotorControlDevRef"=w223) -> ()  [unwired: 7 in, 3 out]
        }
        frame True {
          n83 = call <vilib>:"CTRE_Phoenix_MotorControl_Set.vi"("Output"=w225, "Control Mode"=w233, "PhoenixMotorControlDevRef"=w224) -> ("error out"=w230:errorcluster, "PhoenixMotorControlDevRef"=w231:T19)  [unwired: 7 in]
          n84 = call <vilib>:"CTRE_Phoenix_MotorControl_GetActiveTrajectory.vi"("PhoenixMotorControlDevRef"=w231, "error in"=w230) -> ("Position (Sensor Units)"=w229:i32, "Velocity (Sensor Units per 100 ms)"=w228:i32)  [unwired: 9 in, 3 out]
          n85 = call-poly <vilib>:"CTRE_Phoenix_MotorController_Get_Enhanced.vi"("PhoenixMotorControlDevRef"=w231, "error in"=w230) -> ("Position (Raw Sensor Units)"=w227:i32, "Velocity (Raw Sensor Units per 100 ms)"=w226:i32)  [unwired: 10 in, 2 out]
          n86 = Bundle("Position (Sensor Units)"=w229, "Velocity (Sensor Units per 100 ms)"=w228, "Position (Raw Sensor Units)"=w227, "Velocity (Raw Sensor Units per 100 ms)"=w226) -> (w232:T18)  [unwired: 1 in]
        }
      }
      n87 = case shown="False" w179 {
        tunnel: w176 -> [_ w220]
        tunnel: w194 -> [w209 w219]
        tunnel: [T18 {"Position (Sensor Units)"=0, "Velocity (Sensor Units per 100 ms)"=0, "Position (Raw Sensor Units)"=0, "Velocity (Raw Sensor Units per 100 ms)"=0} w212] -> w189
        tunnel: w182 -> [w210 w211]
        frame False {
          n88 = call "MotorSetInvalidHandler.vi"("Output"=w209, "MotorControlDevRef"=w210) -> ()  [unwired: 7 in, 3 out]
        }
        frame True {
          n89 = call <vilib>:"CTRE_Phoenix_MotorControl_Set.vi"("Output"=w219, "Control Mode"=w220, "PhoenixMotorControlDevRef"=w211) -> ("error out"=w217:errorcluster, "PhoenixMotorControlDevRef"=w218:T19)  [unwired: 7 in]
          n90 = call <vilib>:"CTRE_Phoenix_MotorControl_GetActiveTrajectory.vi"("PhoenixMotorControlDevRef"=w218, "error in"=w217) -> ("Position (Sensor Units)"=w216:i32, "Velocity (Sensor Units per 100 ms)"=w215:i32)  [unwired: 9 in, 3 out]
          n91 = call-poly <vilib>:"CTRE_Phoenix_MotorController_Get_Enhanced.vi"("PhoenixMotorControlDevRef"=w218, "error in"=w217) -> ("Position (Raw Sensor Units)"=w214:i32, "Velocity (Raw Sensor Units per 100 ms)"=w213:i32)  [unwired: 10 in, 2 out]
          n92 = Bundle("Position (Sensor Units)"=w216, "Velocity (Sensor Units per 100 ms)"=w215, "Position (Raw Sensor Units)"=w214, "Velocity (Raw Sensor Units per 100 ms)"=w213) -> (w212:T18)  [unwired: 1 in]
        }
      }
      n93 = case shown="False" w172 {
        tunnel: w176 -> [_ w207]
        tunnel: w177 -> [w196 w206]
        tunnel: [T18 {"Position (Sensor Units)"=0, "Velocity (Sensor Units per 100 ms)"=0, "Position (Raw Sensor Units)"=0, "Velocity (Raw Sensor Units per 100 ms)"=0} w199] -> w175
        tunnel: w178 -> [w197 w198]
        frame False {
          n94 = call "MotorSetInvalidHandler.vi"("Output"=w196, "MotorControlDevRef"=w197) -> ()  [unwired: 7 in, 3 out]
        }
        frame True {
          n95 = call <vilib>:"CTRE_Phoenix_MotorControl_Set.vi"("Output"=w206, "Control Mode"=w207, "PhoenixMotorControlDevRef"=w198) -> ("error out"=w204:errorcluster, "PhoenixMotorControlDevRef"=w205:T19)  [unwired: 7 in]
          n96 = call <vilib>:"CTRE_Phoenix_MotorControl_GetActiveTrajectory.vi"("PhoenixMotorControlDevRef"=w205, "error in"=w204) -> ("Position (Sensor Units)"=w203:i32, "Velocity (Sensor Units per 100 ms)"=w202:i32)  [unwired: 9 in, 3 out]
          n97 = call-poly <vilib>:"CTRE_Phoenix_MotorController_Get_Enhanced.vi"("PhoenixMotorControlDevRef"=w205, "error in"=w204) -> ("Position (Raw Sensor Units)"=w201:i32, "Velocity (Raw Sensor Units per 100 ms)"=w200:i32)  [unwired: 10 in, 2 out]
          n98 = Bundle("Position (Sensor Units)"=w203, "Velocity (Sensor Units per 100 ms)"=w202, "Position (Raw Sensor Units)"=w201, "Velocity (Raw Sensor Units per 100 ms)"=w200) -> (w199:T18)  [unwired: 1 in]
        }
      }
    }
    frame "Auto_Idle", "Auto_Run" {
      # "If arm appears to be stalled,\ncancel auto motion and fall back\ninto manual control"
      # "Tracking and diagnostics"
      n99 = global read "MotionProfileControlData.vi" "ArmShoulderMPControl"() -> (w322:T34)
      n100 = global read "MotionProfileControlData.vi" "ArmExtendMPControl"() -> (w323:T34)
      n101 = global read "MotionProfileControlData.vi" "ArmWristMPControl"() -> (w288:T34)
      n102 = Unbundle By Name(w323) -> ("ControlMutex"=w324:T35)
      n103 = call <vilib>:"Acquire Semaphore.vi"("semaphore"=w324) -> ("error out"=w325:errorcluster, "semaphore out"=w320:T35)  [unwired: 4 in, 1 out]
      n104 = feedback #3() -> (w316:T28)  [unwired: 1 in]
      n105 = flat-sequence {
        tunnel: w348 -> [w429]
        tunnel: w347 -> [w428]
        tunnel: w325 -> [w427]
        tunnel: w328 -> [w426]
        tunnel: w326 -> [w425]
        tunnel: [w424] -> w346
        tunnel: [w423] -> w344
        tunnel: w323 -> [w422]
        tunnel: w322 -> [w421]
        tunnel: w350 -> [w420]
        tunnel: w349 -> [w419]
        tunnel: [w418] -> w321
        tunnel: [w417] -> w343
        tunnel: w320 -> [w416]
        tunnel: [w416] -> w319
        tunnel: w268 -> [w415]
        tunnel: [w414] -> w314
        tunnel: w316 -> [w413]
        tunnel: w315 -> [w412]
        tunnel: [w411] -> w304
        tunnel: w289 -> [w410]
        tunnel: [w409] -> w286
        tunnel: [w408] -> w285
        tunnel: w288 -> [w407]
        tunnel: w287 -> [w406]
        tunnel: w275 -> [w405]
        frame #0 {
          n106 = case shown="\"Commit Points\"" w415 {
            selector: w415 -> [w444 _ w537 w569 w596]
            tunnel: w429 -> [w470 w505 w565 w571 w598]
            tunnel: w428 -> [w469 w504 w564 w570 w597]
            tunnel: w427 -> [_ w486 w526 w567 w579]
            tunnel: w426 -> [_ w513 _ _ _]
            tunnel: w425 -> [_ w512 _ _ _]
            tunnel: [w463 w502 w541 w571 w589] -> w424
            tunnel: [w464 w503 w539 w570 w587] -> w423
            tunnel: w422 -> [w447 w511 _ _ w584]
            tunnel: w421 -> [w446 w497 _ _ w585]
            tunnel: w420 -> [_ w510 _ _ _]
            tunnel: w419 -> [_ w509 _ _ _]
            tunnel: [w462 w500 w540 w567 w588] -> w418
            tunnel: [w461 w501 w538 w567 w586] -> w417
            tunnel: [w454 MPSendState."Enable" ("MP Send State") w554 w569 w596] -> w414
            tunnel: w413 -> [w453 _ w559 _ w595]
            tunnel: w412 -> [w448 _ w558 _ _]
            tunnel: [w442 FALSE FALSE FALSE FALSE] -> w411
            tunnel: w410 -> [w434 w487 w528 w566 w580]
            tunnel: [w431 w488 w525 w566 w572] -> w409
            tunnel: [w430 w489 w524 w567 w573] -> w408
            tunnel: w407 -> [w440 w483 _ _ w576]
            tunnel: w406 -> [_ w485 _ _ _]
            tunnel: w405 -> [_ w490 _ _ _]
            frame "Disable", Default {
              w436 = 0.0 ("Output")
              w435 = T33 6 items=["PercentOutput"=0, "Position"=1, "Velocity"=2, "Current"=3, "Follower"=5, "MotionProfile"=6, "MotionMagic"=7, "MotionMagicArc"=8, "MotionProfileArc"=10, "Disabled"=15] ("Control Mode")
              n107 = First Call?() -> (First Call?: T/F=w441:bool)
              n108 = Not Equal?(x=w444, y=w453) -> (x != y?=w443:bool)
              n109 = Or(x=w443, y=w441) -> (x .or. y?=w442:bool)
              n110 = Tick Count (ms)() -> (millisecond timer value=w451:u32)
              n111 = call <vilib>:"CTRE_Phoenix_MotorControl_Set.vi"("Output"=w436, "Control Mode"=w435, "PhoenixMotorControlDevRef"=w470) -> ("error out"=w473:errorcluster, "PhoenixMotorControlDevRef"=w474:T19)  [unwired: 7 in]
              n112 = call <vilib>:"CTRE_Phoenix_MotorControl_Set.vi"("Output"=w436, "Control Mode"=w435, "PhoenixMotorControlDevRef"=w469) -> ("error out"=w472:errorcluster, "PhoenixMotorControlDevRef"=w471:T19)  [unwired: 7 in]
              n113 = call <vilib>:"CTRE_Phoenix_MotorControl_Set.vi"("Output"=w436, "Control Mode"=w435, "PhoenixMotorControlDevRef"=w434) -> ("error out"=w433:errorcluster, "PhoenixMotorControlDevRef"=w437:T19)  [unwired: 7 in]
              n114 = feedback #4() -> (w452:u32)  [unwired: 1 in]
              n115 = Select(t=w451, s=w442, f=w452) -> (s? t:f=w450:u32)
              n116 = feedback-in #4(w450) -> ()
              n117 = call <vilib>:"CTRE_Phoenix_MotorControl_GetMotionProfileStatus.vi"("error in"=w473, "PhoenixMotorControlDevRef"=w474) -> ("error out"=w462:errorcluster, "Motion Profile Status"=w468:T26, "PhoenixMotorControlDevRef"=w463:T19)  [unwired: 7 in]
              n118 = call <vilib>:"CTRE_Phoenix_MotorControl_GetMotionProfileStatus.vi"("error in"=w472, "PhoenixMotorControlDevRef"=w471) -> ("error out"=w461:errorcluster, "Motion Profile Status"=w467:T26, "PhoenixMotorControlDevRef"=w464:T19)  [unwired: 7 in]
              n119 = call <vilib>:"CTRE_Phoenix_MotorControl_GetMotionProfileStatus.vi"("error in"=w433, "PhoenixMotorControlDevRef"=w437) -> ("error out"=w430:errorcluster, "Motion Profile Status"=w438:T26, "PhoenixMotorControlDevRef"=w431:T19)  [unwired: 7 in]
              n120 = Subtract(x=w451, y=w450) -> (x-y=w449:u32)
              n121 = Unbundle By Name(w468) -> ("Output Enable"=w466:i32)
              n122 = Unbundle By Name(w467) -> ("Output Enable"=w465:i32)
              n123 = Unbundle By Name(w438) -> ("Output Enable"=w439:i32)
              n124 = Greater?(x=w449, y=w448) -> (0:w445:bool)
              n125 = case shown="True" w442 {
                tunnel: w447 -> [_ w481]
                tunnel: w446 -> [_ w480]
                tunnel: w440 -> [_ w479]
                frame False {
                }
                frame True {
                  w475 = u32 0 ("CurrentIndex")
                  w476 = T22[] [] ("Trajectory Points")
                  n126 = Bundle By Name(cluster=w481, "Trajectory Points"=w476, "CurrentIndex"=w475) -> (w482:T34)
                  n127 = Bundle By Name(cluster=w479, "Trajectory Points"=w476, "CurrentIndex"=w475) -> (w477:T34)
                  n128 = Bundle By Name(cluster=w480, "Trajectory Points"=w476, "CurrentIndex"=w475) -> (w478:T34)
                  n129 = global write "MotionProfileControlData.vi" "ArmShoulderMPControl"(w478) -> ()
                  n130 = global write "MotionProfileControlData.vi" "ArmExtendMPControl"(w482) -> ()
                  n131 = global write "MotionProfileControlData.vi" "ArmWristMPControl"(w477) -> ()
                }
              }
              n132 = Equal To 0?(x=w466) -> (x = 0?=w460:bool)
              n133 = Equal To 0?(x=w465) -> (x = 0?=w459:bool)
              n134 = Equal To 0?(x=w439) -> (x = 0?=w432:bool)
              n135 = Compound Arithmetic op=AND(w460, w459, w432) -> (w458:bool)
              n136 = Select(t=MPSendState."Failed", s=w445, f=w444) -> (s? t:f=w457:T28)
              n137 = Select(t=MPSendState."Commit Points", s=w458, f=w457) -> (s? t:f=w454:T28)
            }
            frame "Commit Points" {
              # "Prime motion profiling\nby entering hold mode"
              n138 = call <vilib>:"CTRE_Phoenix_MotorControl_ClearMotionProfileTrajectories.vi"("PhoenixMotorControlDevRef"=w504, "error in"=w486) -> ("PhoenixMotorControlDevRef"=w521:T19, "error out"=w520:errorcluster)  [unwired: 12 in]
              n139 = call <vilib>:"CTRE_Phoenix_MotorControl_ClearMotionProfileTrajectories.vi"("PhoenixMotorControlDevRef"=w487, "error in"=w486) -> ("PhoenixMotorControlDevRef"=w491:T19, "error out"=w492:errorcluster)  [unwired: 12 in]
              n140 = call <vilib>:"CTRE_Phoenix_MotorControl_ClearMotionProfileTrajectories.vi"("PhoenixMotorControlDevRef"=w505, "error in"=w486) -> ("PhoenixMotorControlDevRef"=w519:T19, "error out"=w518:errorcluster)  [unwired: 12 in]
              n141 = call <vilib>:"CTRE_Phoenix_MotorControl_ClearMotionProfileHasUnderrun.vi"("error in"=w518, "PhoenixMotorControlDevRef"=w519) -> ("error out"=w500:errorcluster, "PhoenixMotorControlDevRef"=w517:T19)  [unwired: 8 in]
              n142 = call <vilib>:"CTRE_Phoenix_MotorControl_ClearMotionProfileHasUnderrun.vi"("error in"=w520, "PhoenixMotorControlDevRef"=w521) -> ("error out"=w501:errorcluster, "PhoenixMotorControlDevRef"=w516:T19)  [unwired: 8 in]
              n143 = call <vilib>:"CTRE_Phoenix_MotorControl_ClearMotionProfileHasUnderrun.vi"("error in"=w492, "PhoenixMotorControlDevRef"=w491) -> ("error out"=w489:errorcluster, "PhoenixMotorControlDevRef"=w493:T19)  [unwired: 8 in]
              n144 = call "MotionProfileWriter.vi"("PhoenixMotorControlDevRef"=w517, "Trajectory Points"=w510, "Sensor unit conversion"=w513, "startIndex"=0) -> ("PhoenixMotorControlDevRef Out"=w502:T19, "endIndex"=w508:i32)  [unwired: 10 in]
              n145 = call "MotionProfileWriter.vi"("PhoenixMotorControlDevRef"=w516, "Trajectory Points"=w509, "Sensor unit conversion"=w512, "startIndex"=0) -> ("PhoenixMotorControlDevRef Out"=w503:T19, "endIndex"=w507:i32)  [unwired: 10 in]
              n146 = call "MotionProfileWriter.vi"("PhoenixMotorControlDevRef"=w493, "Trajectory Points"=w485, "Sensor unit conversion"=w490, "startIndex"=0) -> ("PhoenixMotorControlDevRef Out"=w488:T19, "endIndex"=w484:i32)  [unwired: 10 in]
              n147 = Bundle By Name(cluster=w511, "Trajectory Points"=w510, "CurrentIndex"=w508) -> (w506:T34)
              n148 = Bundle By Name(cluster=w497, "Trajectory Points"=w509, "CurrentIndex"=w507) -> (w495:T34)
              n149 = Bundle By Name(cluster=w483, "Trajectory Points"=w485, "CurrentIndex"=w484) -> (w496:T34)
              n150 = global write "MotionProfileControlData.vi" "ArmShoulderMPControl"(w495) -> ()
              n151 = global write "MotionProfileControlData.vi" "ArmExtendMPControl"(w506) -> ()
              n152 = global write "MotionProfileControlData.vi" "ArmWristMPControl"(w496) -> ()
            }
            frame "Enable" {
              w522 = 1.0 ("Output")
              w527 = T33 6 items=["PercentOutput"=0, "Position"=1, "Velocity"=2, "Current"=3, "Follower"=5, "MotionProfile"=6, "MotionMagic"=7, "MotionMagicArc"=8, "MotionProfileArc"=10, "Disabled"=15] ("Control Mode")
              # "Transition to execute mode"
              n153 = Not Equal?(x=w537, y=w559) -> (x != y?=w534:bool)
              n154 = First Call?() -> (First Call?: T/F=w533:bool)
              n155 = Tick Count (ms)() -> (millisecond timer value=w562:u32)
              n156 = Or(x=w534, y=w533) -> (x .or. y?=w535:bool)
              n157 = feedback #5() -> (w563:u32)  [unwired: 1 in]
              n158 = Select(t=w562, s=w535, f=w563) -> (s? t:f=w561:u32)
              n159 = feedback-in #5(w561) -> ()
              n160 = Subtract(x=w562, y=w561) -> (x-y=w560:u32)
              n161 = Greater?(x=w560, y=w558) -> (0:w553:bool)
              n162 = call <vilib>:"CTRE_Phoenix_MotorControl_Set.vi"("error in (no error)"=w526, "Output"=w522, "Control Mode"=w527, "PhoenixMotorControlDevRef"=w528) -> ("error out"=w531:errorcluster, "PhoenixMotorControlDevRef"=w530:T19)  [unwired: 6 in]
              n163 = call <vilib>:"CTRE_Phoenix_MotorControl_Set.vi"("error in (no error)"=w526, "Output"=w522, "Control Mode"=w527, "PhoenixMotorControlDevRef"=w564) -> ("error out"=w547:errorcluster, "PhoenixMotorControlDevRef"=w548:T19)  [unwired: 6 in]
              n164 = call <vilib>:"CTRE_Phoenix_MotorControl_Set.vi"("error in (no error)"=w526, "Output"=w522, "Control Mode"=w527, "PhoenixMotorControlDevRef"=w565) -> ("error out"=w545:errorcluster, "PhoenixMotorControlDevRef"=w546:T19)  [unwired: 6 in]
              n165 = call <vilib>:"CTRE_Phoenix_MotorControl_GetMotionProfileStatus.vi"("error in"=w531, "PhoenixMotorControlDevRef"=w530) -> ("error out"=w524:errorcluster, "Motion Profile Status"=w529:T26, "PhoenixMotorControlDevRef"=w525:T19)  [unwired: 7 in]
              n166 = call <vilib>:"CTRE_Phoenix_MotorControl_GetMotionProfileStatus.vi"("error in"=w545, "PhoenixMotorControlDevRef"=w546) -> ("error out"=w540:errorcluster, "Motion Profile Status"=w552:T26, "PhoenixMotorControlDevRef"=w541:T19)  [unwired: 7 in]
              n167 = call <vilib>:"CTRE_Phoenix_MotorControl_GetMotionProfileStatus.vi"("error in"=w547, "PhoenixMotorControlDevRef"=w548) -> ("error out"=w538:errorcluster, "Motion Profile Status"=w551:T26, "PhoenixMotorControlDevRef"=w539:T19)  [unwired: 7 in]
              n168 = Unbundle By Name(w529) -> ("Output Enable"=w532:i32)
              n169 = Unbundle By Name(w552) -> ("Output Enable"=w544:i32)
              n170 = Unbundle By Name(w551) -> ("Output Enable"=w543:i32)
              n171 = Equal?(x=w532, y=w522) -> (x = y?=w523:bool)
              n172 = Equal?(x=w544, y=w522) -> (x = y?=w550:bool)
              n173 = Equal?(x=w543, y=w522) -> (x = y?=w549:bool)
              n174 = Compound Arithmetic op=AND(w550, w549, w523) -> (w542:bool)
              n175 = Select(t=MPSendState."Failed", s=w553, f=w537) -> (s? t:f=w557:T28)
              n176 = Select(t=MPSendState."Done", s=w542, f=w557) -> (s? t:f=w554:T28)
            }
            frame "Done" {
            }
            frame "Failed" {
              w577 = 0.0 ("Output")
              w578 = T33 6 items=["PercentOutput"=0, "Position"=1, "Velocity"=2, "Current"=3, "Follower"=5, "MotionProfile"=6, "MotionMagic"=7, "MotionMagicArc"=8, "MotionProfileArc"=10, "Disabled"=15] ("Control Mode")
              n177 = Not Equal?(x=w596, y=w595) -> (x != y?=w594:bool)
              n178 = First Call?() -> (First Call?: T/F=w581:bool)
              n179 = Or(x=w594, y=w581) -> (x .or. y?=w582:bool)
              n180 = call <vilib>:"CTRE_Phoenix_MotorControl_Set.vi"("error in (no error)"=w579, "Output"=w577, "Control Mode"=w578, "PhoenixMotorControlDevRef"=w598) -> ("error out"=w591:errorcluster, "PhoenixMotorControlDevRef"=w593:T19)  [unwired: 6 in]
              n181 = call <vilib>:"CTRE_Phoenix_MotorControl_Set.vi"("error in (no error)"=w579, "Output"=w577, "Control Mode"=w578, "PhoenixMotorControlDevRef"=w597) -> ("error out"=w590:errorcluster, "PhoenixMotorControlDevRef"=w592:T19)  [unwired: 6 in]
              n182 = call <vilib>:"CTRE_Phoenix_MotorControl_Set.vi"("error in (no error)"=w579, "Output"=w577, "Control Mode"=w578, "PhoenixMotorControlDevRef"=w580) -> ("error out"=w574:errorcluster, "PhoenixMotorControlDevRef"=w575:T19)  [unwired: 6 in]
              n183 = case shown="True" w582 {
                tunnel: w593 -> [w604 w624]
                tunnel: w592 -> [w602 w622]
                tunnel: w591 -> [w603 w623]
                tunnel: w590 -> [w601 w621]
                tunnel: [w604 w620] -> w589
                tunnel: [w603 w619] -> w588
                tunnel: [w602 w618] -> w587
                tunnel: [w601 w617] -> w586
                tunnel: w585 -> [_ w613]
                tunnel: w584 -> [_ w615]
                tunnel: w576 -> [_ w609]
                tunnel: w575 -> [w600 w608]
                tunnel: w574 -> [w599 w607]
                tunnel: [w599 w606] -> w573
                tunnel: [w600 w605] -> w572
                frame False {
                }
                frame True {
                  w610 = u32 0 ("CurrentIndex")
                  w611 = T22[] [] ("Trajectory Points")
                  n184 = call <vilib>:"CTRE_Phoenix_MotorControl_ClearMotionProfileTrajectories.vi"("PhoenixMotorControlDevRef"=w608, "error in"=w607) -> ("PhoenixMotorControlDevRef"=w605:T19, "error out"=w606:errorcluster)  [unwired: 12 in]
                  n185 = call <vilib>:"CTRE_Phoenix_MotorControl_ClearMotionProfileTrajectories.vi"("PhoenixMotorControlDevRef"=w624, "error in"=w623) -> ("PhoenixMotorControlDevRef"=w620:T19, "error out"=w619:errorcluster)  [unwired: 12 in]
                  n186 = call <vilib>:"CTRE_Phoenix_MotorControl_ClearMotionProfileTrajectories.vi"("PhoenixMotorControlDevRef"=w622, "error in"=w621) -> ("PhoenixMotorControlDevRef"=w618:T19, "error out"=w617:errorcluster)  [unwired: 12 in]
                  n187 = Bundle By Name(cluster=w615, "Trajectory Points"=w611, "CurrentIndex"=w610) -> (w616:T34)
                  n188 = Bundle By Name(cluster=w613, "Trajectory Points"=w611, "CurrentIndex"=w610) -> (w614:T34)
                  n189 = Bundle By Name(cluster=w609, "Trajectory Points"=w611, "CurrentIndex"=w610) -> (w612:T34)
                  n190 = global write "MotionProfileControlData.vi" "ArmShoulderMPControl"(w614) -> ()
                  n191 = global write "MotionProfileControlData.vi" "ArmExtendMPControl"(w616) -> ()
                  n192 = global write "MotionProfileControlData.vi" "ArmWristMPControl"(w612) -> ()
                }
              }
            }
          }
        }
      }
      n193 = feedback-in #6(w314) -> ()
      n194 = feedback #6() -> (w317:T28)  [unwired: 1 in]
      n195 = Select(t=MPSendState."Disable" ("MP Send State"), s=w298, f=w317) -> (s? t:f=w268:T28)
      n196 = global write "DriversStationData.vi" "Arm MP Send State"(w268) -> ()
      n197 = feedback-in #3(w268) -> ()
      n198 = call <vilib>:"Release Semaphore.vi"("error in (no error)"=w321, "semaphore"=w319) -> ("error out"=w345:errorcluster)  [unwired: 4 in, 1 out]
      n199 = feedback #7(errorcluster {"status"=FALSE, "code"=0, "source"=""} ("error IO")) -> (w301:errorcluster)
      n200 = Compound Arithmetic op=AND(invert w301, w304) -> (w303:bool)
      n201 = case shown="True" w303 {
        tunnel: [w392 w400] -> w309
        tunnel: [w392 w399] -> w308
        tunnel: [w392 w398] -> w307
        tunnel: [w392 w397] -> w306
        tunnel: w301 -> [w392 _]
        tunnel: [w392 w394] -> w297
        tunnel: [w392 w393] -> w296
        frame False {
        }
        frame True {
          # "Reset plots"
          n202 = property on="ArmExtension" class="WFChart (strict)"("History Data"=T32 []) -> (error out=w400:errorcluster)  [unwired: 2 in, 1 out]
          n203 = property on="ArmShoulder" class="WFChart (strict)"("History Data"=T32 []) -> (error out=w398:errorcluster)  [unwired: 2 in, 1 out]
          n204 = property on="ArmShoulderV" class="WFChart (strict)"("History Data"=dbl[] []) -> (error out=w397:errorcluster)  [unwired: 2 in, 1 out]
          n205 = property on="ArmWrist" class="WFChart (strict)"("History Data"=T32 []) -> (error out=w394:errorcluster)  [unwired: 2 in, 1 out]
          n206 = property on="ArmExtensionV" class="WFChart (strict)"("History Data"=dbl[] []) -> (error out=w399:errorcluster)  [unwired: 2 in, 1 out]
          n207 = property on="ArmWristV" class="WFChart (strict)"("History Data"=dbl[] []) -> (error out=w393:errorcluster)  [unwired: 2 in, 1 out]
        }
      }
      n208 = Merge Errors(w309, w308, w307, w306, w297, w296) -> (w305:errorcluster)
      n209 = feedback-in #7(w305) -> ()
      n210 = call-poly <vilib>:"CTRE_Phoenix_MotorController_Get_Enhanced.vi"("PhoenixMotorControlDevRef"=w346, "error in"=w345) -> ("Output Voltage"=w367:dbl)  [unwired: 9 in, 4 out]
      n211 = call-poly <vilib>:"CTRE_Phoenix_MotorController_Get_Enhanced.vi"("PhoenixMotorControlDevRef"=w344, "error in"=w343) -> ("Output Voltage"=w368:dbl)  [unwired: 9 in, 4 out]
      n212 = call-poly <vilib>:"CTRE_Phoenix_MotorController_Get_Enhanced.vi"("PhoenixMotorControlDevRef"=w286, "error in"=w285) -> ("Output Voltage"=w284:dbl)  [unwired: 9 in, 4 out]
      n213 = call <vilib>:"CTRE_Phoenix_MotorControl_GetMotionProfileStatus.vi"("error in"=w345, "PhoenixMotorControlDevRef"=w346) -> ("Motion Profile Status"=w362:T26)  [unwired: 7 in, 2 out]
      n214 = call <vilib>:"CTRE_Phoenix_MotorControl_GetActiveTrajectory.vi"("PhoenixMotorControlDevRef"=w346, "error in"=w345) -> ("Position (Sensor Units)"=w388:i32, "Velocity (Sensor Units per 100 ms)"=w387:i32)  [unwired: 9 in, 3 out]
      n215 = call-poly <vilib>:"CTRE_Phoenix_MotorController_Get_Enhanced.vi"("PhoenixMotorControlDevRef"=w346, "error in"=w345) -> ("Position (Raw Sensor Units)"=w386:i32, "Velocity (Raw Sensor Units per 100 ms)"=w370:i32)  [unwired: 10 in, 2 out]
      n216 = call <vilib>:"CTRE_Phoenix_MotorControl_GetMotionProfileStatus.vi"("error in"=w343, "PhoenixMotorControlDevRef"=w344) -> ("Motion Profile Status"=w363:T26)  [unwired: 7 in, 2 out]
      n217 = call <vilib>:"CTRE_Phoenix_MotorControl_GetActiveTrajectory.vi"("PhoenixMotorControlDevRef"=w344, "error in"=w343) -> ("Position (Sensor Units)"=w385:i32, "Velocity (Sensor Units per 100 ms)"=w384:i32)  [unwired: 9 in, 3 out]
      n218 = call-poly <vilib>:"CTRE_Phoenix_MotorController_Get_Enhanced.vi"("PhoenixMotorControlDevRef"=w344, "error in"=w343) -> ("Position (Raw Sensor Units)"=w383:i32, "Velocity (Raw Sensor Units per 100 ms)"=w373:i32)  [unwired: 10 in, 2 out]
      n219 = call <vilib>:"CTRE_Phoenix_MotorControl_GetMotionProfileStatus.vi"("error in"=w285, "PhoenixMotorControlDevRef"=w286) -> ("Motion Profile Status"=w283:T26)  [unwired: 7 in, 2 out]
      n220 = call <vilib>:"CTRE_Phoenix_MotorControl_GetActiveTrajectory.vi"("PhoenixMotorControlDevRef"=w286, "error in"=w285) -> ("Position (Sensor Units)"=w290:i32, "Velocity (Sensor Units per 100 ms)"=w291:i32)  [unwired: 9 in, 3 out]
      n221 = call-poly <vilib>:"CTRE_Phoenix_MotorController_Get_Enhanced.vi"("PhoenixMotorControlDevRef"=w286, "error in"=w285) -> ("Position (Raw Sensor Units)"=w292:i32, "Velocity (Raw Sensor Units per 100 ms)"=w294:i32)  [unwired: 10 in, 2 out]
      n222 = Unbundle By Name(w363) -> ("Output Enable"=w376:i32, "Is Last?"=w340:bool)
      n223 = Unbundle By Name(w283) -> ("Output Enable"=w273:i32, "Is Last?"=w272:bool)
      n224 = Unbundle By Name(w362) -> ("Output Enable"=w382:i32, "Is Last?"=w339:bool)
      n225 = Multiply(x=w370, y=10) -> (x*y=w371:i32)
      n226 = Multiply(x=w373, y=10) -> (x*y=w374:i32)
      n227 = Multiply(x=w294, y=10) -> (x*y=w293:i32)
      n228 = Bundle("Position (Sensor Units)"=w388, "Velocity (Sensor Units per 100 ms)"=w387, "Position (Raw Sensor Units)"=w386, w371) -> (w338:T36)  [unwired: 1 in]
      n229 = Bundle("Position (Sensor Units)"=w385, "Velocity (Sensor Units per 100 ms)"=w384, "Position (Raw Sensor Units)"=w383, w374) -> (w337:T36)  [unwired: 1 in]
      n230 = Bundle("Position (Sensor Units)"=w290, "Velocity (Sensor Units per 100 ms)"=w291, "Position (Raw Sensor Units)"=w292, w293) -> (w269:T36)  [unwired: 1 in]
      n231 = Equal?(x=1, y=w273) -> (x = y?=w271:bool)
      n232 = Equal?(x=1, y=w382) -> (x = y?=w380:bool)
      n233 = Equal?(x=1, y=w376) -> (x = y?=w378:bool)
      n234 = Compound Arithmetic op=AND(w340, w339, w272) -> (w313:bool)
      n235 = Compound Arithmetic op=AND(w271, invert w272) -> (w270:bool)
      n236 = Unbundle(w338) -> ("Position (Sensor Units)"=w336:i32, "Position (Raw Sensor Units)"=w335:i32)  [unwired: 2 out]
      n237 = Unbundle(w269) -> ("Position (Sensor Units)"=w280:i32, "Position (Raw Sensor Units)"=w281:i32)  [unwired: 2 out]
      n238 = Unbundle(w337) -> ("Position (Sensor Units)"=w334:i32, "Position (Raw Sensor Units)"=w333:i32)  [unwired: 2 out]
      n239 = Compound Arithmetic op=AND(w380, invert w339) -> (w379:bool)
      n240 = Compound Arithmetic op=AND(w378, invert w340) -> (w375:bool)
      n241 = call "EdgeDetector.vi"("DetectorType"=EdgeDetector_Type."RisingEdge", "Input"=w313) -> ("Edge"=w311:bool)
      n242 = Subtract(x=w280, y=w281) -> (x-y=w279:i32)
      n243 = Subtract(x=w334, y=w333) -> (x-y=w341:i32)
      n244 = Subtract(x=w336, y=w335) -> (x-y=w342:i32)
      n245 = Absolute Value(x=w279) -> (abs(x)=w282:i32)
      n246 = Absolute Value(x=w341) -> (abs(x)=w327:i32)
      n247 = Absolute Value(x=w342) -> (abs(x)=w329:i32)
      n248 = Divide(x=w282, y=w275) -> (x/y=w278:dbl)
      n249 = Divide(x=w329, y=w328) -> (x/y=w361:dbl)
      n250 = Divide(x=w327, y=w326) -> (x/y=w360:dbl)
      n251 = Greater?(x=w278, y=w276) -> (0:w277:bool)
      n252 = Greater?(x=w361, y=w358) -> (0:w357:bool)
      n253 = Greater?(x=w360, y=w359) -> (0:w356:bool)
      n254 = case shown="True" w311 {
        selector: w311 -> [_ w391]
        tunnel: "ArmCompleteNotifier" -> [_ w390]
        frame False {
        }
        frame True {
          n255 = Send Notification(notification=w391, notifier=w390) -> ()  [unwired: 1 in, 2 out]
        }
      }
      n256 = call "Timed_DeBounce.vi"("Input"=w357, "Reset"=w298, "Hold Time(ms)"=w300) -> ("Output"=w355:bool)
      n257 = call "Timed_DeBounce.vi"("Input"=w356, "Reset"=w298, "Hold Time(ms)"=w300) -> ("Output"=w354:bool)
      n258 = call "Timed_DeBounce.vi"("Input"=w277, "Reset"=w298, "Hold Time(ms)"=w300) -> ("Output"=w299:bool)
      n259 = feedback #8() -> (w364:T24)  [unwired: 1 in]
      n260 = Select(t=MotionProfileControlState."Auto_Run" ("Arm Control State"), s=w298, f=w364) -> (s? t:f=w365:T24)
      n261 = Select(t=MotionProfileControlState."Auto_Idle" ("Arm Control State"), s=w313, f=w365) -> (s? t:f=w352:T24)
      n262 = Compound Arithmetic op=OR(w355, w354, w299) -> (w332:bool)
      n263 = And(x=w332, y=w330) -> (x .and. y?=w331:bool)
      n264 = Select(t=MotionProfileControlState."Manual", s=w331, f=w352) -> (s? t:f=w353:T24)
      n265 = feedback-in #8(w353) -> ()
      "MP Send State" <- w314
    }
  }
  "Arm Control State" <- w74
  "Extension" <- w125
  "ShoulderRotate" <- w124
  "ShoulderRotate" <- w103
  "Extension" <- w102
  "WristRotate" <- w47
  "WristRotate" <- w23
  n266 = feedback-in #2(w74) -> ()
  n267 = Build Array(WPI_DriverStationRobotMode2."Teleop Enabled" ("Robot Mode"), WPI_DriverStationRobotMode2."Autonomous Enabled" ("Robot Mode")) -> (w79:T31[])
  n268 = call <vilib>:"WPI_DriverStationGetModeAndStatus.vi"() -> ("Robot Mode"=w83:T31)  [unwired: 10 in, 1 out]
  n269 = Equal?(x=w79, y=w83) -> (x = y?=w82:bool[])
  n270 = Unbundle By Name(w124) -> ("Velocity (Sensor Units per 100 ms)"=w106:i32, "Position (Raw Sensor Units)"=w137:i32)
  n271 = Unbundle By Name(w23) -> ("Velocity (Sensor Units per 100 ms)"=w42:i32, "Position (Raw Sensor Units)"=w41:i32)
  n272 = Unbundle By Name(w125) -> ("Velocity (Sensor Units per 100 ms)"=w109:i32, "Position (Raw Sensor Units)"=w138:i32)
  n273 = Or Array Elements(Boolean array=w82) -> (logical OR=w45:bool)
  n274 = And(x=w45, y=w143) -> (x .and. y?=w100:bool)
  n275 = And(x=w45, y=w145) -> (x .and. y?=w99:bool)
  n276 = And(x=w45, y=w46) -> (x .and. y?=w34:bool)
  n277 = Divide(x=w138, y="Extend Sensor Unit Coversion (ticks/in)") -> (x/y=w136:dbl)
  n278 = Divide(x=w137, y="Shoulder Sensor Unit Conversion (ticks/rad)") -> (x/y=w135:dbl)
  n279 = Divide(x=w41, y="Wrist Sensor Unit Coversion (ticks/rad)") -> (x/y=w39:dbl)
  n280 = call "CoordinateConvert_ArmToCartesian.vi"("Wrist Angle (rad)"=w39, "Radius (in)"=w136, "Shoulder Angle (rad)"=w135) -> ("Wrist (rad)"=w19:dbl, "Y (in)"=w20:dbl, "X (in)"=w21:dbl)
  n281 = call "HistoricMaxMagnitude.vi"("Reset"="Reset Wrist Rotate Max", "Value"=w42) -> ("Max"=→"Max Wrist Rotate Speed (Sensor Units per 100 ms)":dbl)
  n282 = call "HistoricMaxMagnitude.vi"("Reset"="Reset Extend Max", "Value"=w109) -> ("Max"=→"Max Extend Speed (Sensor Units per 100 ms)":dbl)
  n283 = call "HistoricMaxMagnitude.vi"("Reset"="Reset Shoulder Rotate Max", "Value"=w106) -> ("Max"=→"Max Shoulder Rotate Speed (Sensor Units per 100 ms)":dbl)
  n284 = case shown="True" w100 {
    tunnel: w125 -> [_ w626]
    tunnel: w141 -> [_ w625]
    frame False {
    }
    frame True {
      "ArmExtension" <- w626
      "ArmExtensionV" <- w625
    }
  }
  n285 = case shown="True" w99 {
    tunnel: w124 -> [_ w628]
    tunnel: w142 -> [_ w627]
    frame False {
    }
    frame True {
      "ArmShoulder" <- w628
      "ArmShoulderV" <- w627
    }
  }
  n286 = case shown="True" w34 {
    tunnel: w23 -> [_ w630]
    tunnel: w36 -> [_ w629]
    frame False {
    }
    frame True {
      "ArmWristV" <- w629
      "ArmWrist" <- w630
    }
  }
  n287 = Compound Arithmetic op=OR(w100, w99, w34) -> (w96:bool)
  n288 = call "EdgeDetector.vi"("DetectorType"=EdgeDetector_Type."RisingEdge", "Input"=w96) -> ("Edge"=w84:bool)
  n289 = Bundle By Name(cluster=T30 {"X (in)"=0.0, "Y (in)"=0.0, "Wrist (rad)"=0.0} ("ArmAbsolutePose"), "X (in)"=w21, "Y (in)"=w20, "Wrist (rad)"=w19) -> (w18:T30)
  n290 = feedback #9() -> (w94:dbl[])  [unwired: 1 in]
  n291 = Select(t=w89, s=w84, f=w94) -> (s? t:f=w93:dbl[])
  n292 = feedback #10() -> (w85:cluster{dbl[], dbl[]})  [unwired: 1 in]
  n293 = case shown="True" w84 {
    tunnel: "Arm Extend Motion Profile" -> [_ w637]
    tunnel: "Arm Shoulder Motion Profile" -> [_ w636]
    tunnel: [w631 w633] -> w86
    tunnel: w85 -> [w631 _]
    tunnel: "Arm Wrist Motion Profile" -> [_ w632]
    frame False {
    }
    frame True {
      n294 = for {
        tunnel: w637 -> [w645] mode=indexing
        tunnel: w636 -> [w644] mode=indexing
        tunnel: [w641] -> w635 mode=indexing
        tunnel: [w640] -> w634 mode=indexing
        tunnel: w632 -> [w639] mode=indexing
        n295 = Unbundle By Name(w645) -> ("Position"=w643:dbl)
        n296 = Unbundle By Name(w644) -> ("Position"=w642:dbl)
        n297 = Unbundle By Name(w639) -> ("Position"=w638:dbl)
        n298 = call "CoordinateConvert_ArmToCartesian.vi"("Wrist Angle (rad)"=w638, "Radius (in)"=w643, "Shoulder Angle (rad)"=w642) -> ("Y (in)"=w640:dbl, "X (in)"=w641:dbl)  [unwired: 1 out]
      }
      n299 = Bundle(w635, w634) -> (w633:cluster{dbl[], dbl[]})  [unwired: 1 in]
    }
  }
  n300 = feedback-in #10(w86) -> ()
  n301 = feedback #11() -> (w90:dbl[])  [unwired: 1 in]
  n302 = Select(t=w89, s=w84, f=w90) -> (s? t:f=w92:dbl[])
  n303 = case shown="False" w96 {
    tunnel: w21 -> [_ w653]
    tunnel: w20 -> [_ w652]
    tunnel: [w646 w651] -> w97
    tunnel: [w647 w650] -> w91
    tunnel: w93 -> [w646 w649]
    tunnel: w92 -> [w647 w648]
    frame False {
    }
    frame True {
      n304 = Build Array (concatenate)(w648, w653) -> (w650:dbl[])
      n305 = Build Array (concatenate)(w649, w652) -> (w651:dbl[])
    }
  }
  n306 = feedback-in #9(w97) -> ()
  n307 = feedback-in #11(w91) -> ()
  n308 = global write "DriversStationData.vi" "Arm Position"(w18) -> ()
  n309 = Build Array(w123, w21) -> (w134:dbl[])
  n310 = Build Array(w123, w20) -> (w133:dbl[])
  n311 = Bundle("t"=w91, "t"=w97) -> (w98:cluster{"t":dbl[], "t":dbl[]})  [unwired: 1 in]
  n312 = Bundle(w134, w133) -> (w132:cluster{dbl[], dbl[]})  [unwired: 1 in]
  n313 = Build Array(w86, w98, w132) -> (→"Arm Tracking":cluster{"t":dbl[], "t":dbl[]}[])
